vi "Steuerprogramm09-15.vi"() -> ()   [LabVIEW 2010]
uses:
  <vilib>/rvi/interface/nirviReadWriteControl/nirviReadWriteControl.xnode
  <vilib>/rvi/errors/niLvFpgaWhatHappensToTopLevelVI.ctl
  <vilib>/rvi/interface/common/niFpgaNodeNameForErrorReporting.ctl
  <vilib>/rvi/errors/niLvFpgaAdjustHostInterfaceError.vi
  gvbooleschRT.vi
  <vilib>/functionblocks/FB Core/FB Core.xnode
  <vilib>/functionblocks/Counter/Elapsed Timer/Elapsed Timer.vi
  <vilib>/functionblocks/NI_FunctionBlock Libraries.lvlib
  <vilib>/rvi/interface/nirviCloseFPGA/nirviCloseFPGA.xnode
  <vilib>/addons/control/pid/NI_PID_pid.lvlib
  C:/Users/HAGAR-IV/Desktop/Zeugs/Johnny/pertrasgc fpga/FPGA-Programm-10-14.vi
  C:/Users/HAGAR-IV/Desktop/Zeugs/markus/version feb 2012/FPGA Bitfiles/pertrasgcfpga2_FPGATarget_FPGA-Programm-10_16368CB6.lvbitx
  GVMWHorst.vi
  GVMethodenwechsel.vi
  GVHorstSP.vi
  GVZwangs.vi
  GVHK1Hz.vi
  GVHeizenLH.vi
  GVAIs.vi
  <vilib>/addons/control/pid/pid.llb/PID (DBL Array).vi
  GVTrapsMachs.vi
  GVaktuelleTDMS.vi
  GVECDs.vi
  GVZeitenZyklen.vi
  GVProbenvol.vi
  GVVentilposition.vi
  NiFpgaLv.dll
  <vilib>/Utility/error.llb/Error Cluster From Error Code.vi
  <vilib>/Instr/_visa.llb/VISA Configure Serial Port (Instr).vi
  <vilib>/rvi/interface/nirviMethod/nirviMethod.xnode
  GVChroms.vi
  <vilib>/FPGAPlugInAG/cRIO-9114/niLvFpga_Close_cRIO-9114.vi
panel:
  in  "An/Aus":bool
  in  "dargestellte Größe 3":i32(ring)=1 items=["U_WiderstandTrap1 [V]", "TemperaturTrap1 [°C]", "U_WiderstandTrap2 [V]", "TemperaturTrap2 [°C]", "TemperaturMach1 [°C]", "TemperaturMach2 [°C]", "PrC0", "PrC2C", "Regler18", "Regler17", "Regler19", "Regler16", "Regler15", "Regler14", "MFC2A", "MFC2B", "MFC2C", "PrC2A", "MFC2D", "MFC2E", "PrC2B"]
  in  "TafelWischen!":bool
  out "schnelleAnzeige":cluster{dbl[], dbl[]}(graph)
  in  "senden":bool
  in  "Schreibpuffer":string
  out "vomLicor":string
  in  "Licor":bool
  in  "SerielleKomm.":bool=TRUE
  in  "ECDSpeichern":bool=TRUE
  in  "HKSpeichern":bool
  in  "Methode speichern":bool
  in  "DetYMax":dbl=100.0
  in  "DetYMin":dbl
  in  "HK2YMax":dbl=100.0
  in  "HK2YMin":dbl
  in  "HK1YMax":dbl=100.0
  in  "HK1YMin":dbl
  out "ZyklusNummernGesamt":i32[](array[numeric])
  in  "Detektor":i32(ring) items=["ECD1", "ECD2"]
  out "Detektor":cluster{dbl[], dbl[]}[](graph)
  out "Zykluslängen [s]":dbl[](array[numeric])
  in  "veränderte Methode benutzen":bool
  in  "Methode verändern":bool
  in  "dargestellte Größe 2":i32(ring)=1 items=["T1-Trap1", "T1-Trap2", "T1-Stirling", "T1-PreCol1", "T1-PreCol2", "T1-MainCol1a", "T1-MainCol1b", "T1-MainCol2a", "T1-MainCol2b", "T1-Spare1", "T1-Spare2", "T1-Spare3", "T1-Spare4", "T1-Valve1B", "T1-Spare9", "T1-Valve1A", "T1-Spare10", "T1-TurboPump", "T1-StirlingPlatine", "T1-Spare5", "T1-Spare6", "T1-Spare7", "T1-Spare8", "F1-MFM1", "F1-MFM2", "P1-MethaneHP", "P1-MethaneLP", "P1-Vacuum", "TurboSpeed", "I1-MS-AC", "I1-Trap1", "I1-Trap2", "T2-ECD1a", "T2-ECD1b", "T2-ECD2a", "T2-ECD2b", "T2-Col1a", "T2-Col1b", "T2-Col2a", "T2-Col2b", "T2-Spare1", "T2-Spare2", "T2-Oven_a", "T2-Oven_b", "T2-Spare3", "T2-Spare4", "T2-Spare5", "F2-MFM0", "F2-MFM2A", "F2-MFM2B", "P2-N2O_HP", "P2-N2O_LP", "P2-CO2_HP", "P2-CO2_LP", "AI-Spare1", "AI-Spare2", "AI-Spare3", "AI-Spare4", "AI-Spare5", "AI-Spare6", "AI-Spare7", "AI-Spare8", "AI-Spare9", "AI-Spare10", "T0-DC/DC5", "I0-24V_M0", "I0-48V_M1", "I0-24V_M1", "I0-28V_M2", "T0-Drier", "T0-Spare2", "T0-Spare4", "T0-DC/DC7", "I0-20V_Laptop", "I0-28V_M1", "I0-24V_M2", "I0-12V_Licor", "T0-Spare1", "T0-Spare3", "T0-Spare5", "F0-MFM1", "TL-Licor_a", "P0-NitrogenHP", "P0-HeliumHP", "P0-Standard1HP", "P0-Standard2HP", "P0-Standard3HP", "AI-Spare11", "F0-MFM2", "TL-Licor_b", "P0-NitrogenLP", "P0-HeliumLP", "P0-Standard1LP", "P0-Standard2LP", "P0-Standard3LP", "AI-Spare12", "U_WiderstandTrap1 [V]", "TemperaturTrap1 [°C]", "U_WiderstandTrap2 [V]", "TemperaturTrap2 [°C]", "TemperaturMach1 [°C]", "TemperaturMach2 [°C]", "PrC0", "PrC2C", "Regler18", "Regler17", "Regler19", "Regler16", "Regler15", "Regler14", "MFC2A", "MFC2B", "MFC2C", "PrC2A", "MFC2D", "MFC2E", "PrC2B"]
  in  "Zeitachse2":i32(ring)=1 items=["Zykluszeit [s] Mod0", "Zykluszeit [s] Mod1", "Zykluszeit [s] Mod2A", "Zykluszeit [s] Mod2B"]
  out "Housekeeping2":cluster{dbl[], dbl[]}(graph)
  out "ZyklusNummern":i32[](array[numeric])
  in  "dargestellte Größe 1":i32(ring)=1 items=["T1-Trap1", "T1-Trap2", "T1-Stirling", "T1-PreCol1", "T1-PreCol2", "T1-MainCol1a", "T1-MainCol1b", "T1-MainCol2a", "T1-MainCol2b", "T1-Spare1", "T1-Spare2", "T1-Spare3", "T1-Spare4", "T1-Valve1B", "T1-Spare9", "T1-Valve1A", "T1-Spare10", "T1-TurboPump", "T1-StirlingPlatine", "T1-Spare5", "T1-Spare6", "T1-Spare7", "T1-Spare8", "F1-MFM1", "F1-MFM2", "P1-MethaneHP", "P1-MethaneLP", "P1-Vacuum", "TurboSpeed", "I1-MS-AC", "I1-Trap1", "I1-Trap2", "T2-ECD1a", "T2-ECD1b", "T2-ECD2a", "T2-ECD2b", "T2-Col1a", "T2-Col1b", "T2-Col2a", "T2-Col2b", "T2-Spare1", "T2-Spare2", "T2-Oven_a", "T2-Oven_b", "T2-Spare3", "T2-Spare4", "T2-Spare5", "F2-MFM0", "F2-MFM2A", "F2-MFM2B", "P2-N2O_HP", "P2-N2O_LP", "P2-CO2_HP", "P2-CO2_LP", "AI-Spare1", "AI-Spare2", "AI-Spare3", "AI-Spare4", "AI-Spare5", "AI-Spare6", "AI-Spare7", "AI-Spare8", "AI-Spare9", "AI-Spare10", "T0-DC/DC5", "I0-24V_M0", "I0-48V_M1", "I0-24V_M1", "I0-28V_M2", "T0-Drier", "T0-Spare2", "T0-Spare4", "T0-DC/DC7", "I0-20V_Laptop", "I0-28V_M1", "I0-24V_M2", "I0-12V_Licor", "T0-Spare1", "T0-Spare3", "T0-Spare5", "F0-MFM1", "TL-Licor_a", "P0-NitrogenHP", "P0-HeliumHP", "P0-Standard1HP", "P0-Standard2HP", "P0-Standard3HP", "AI-Spare11", "F0-MFM2", "TL-Licor_b", "P0-NitrogenLP", "P0-HeliumLP", "P0-Standard1LP", "P0-Standard2LP", "P0-Standard3LP", "AI-Spare12", "U_WiderstandTrap1 [V]", "TemperaturTrap1 [°C]", "U_WiderstandTrap2 [V]", "TemperaturTrap2 [°C]", "TemperaturMach1 [°C]", "TemperaturMach2 [°C]", "PrC0", "PrC2C", "Regler18", "Regler17", "Regler19", "Regler16", "Regler15", "Regler14", "MFC2A", "MFC2B", "MFC2C", "PrC2A", "MFC2D", "MFC2E", "PrC2B"]
  in  "Zeitachse1":i32(ring)=1 items=["Zykluszeit [s] Mod0", "Zykluszeit [s] Mod1", "Zykluszeit [s] Mod2A", "Zykluszeit [s] Mod2B"]
  out "Housekeeping1":cluster{dbl[], dbl[]}(graph)
  out "Big Ben, Methodenzeit, Zykluszeit0, Zykluszeit1, Zykluszeit2A, Zykluszeit2B":i32[](array[numeric])
  in  "global stop RT":bool
  in  "Methode":i32(ring) items=["Leer"]
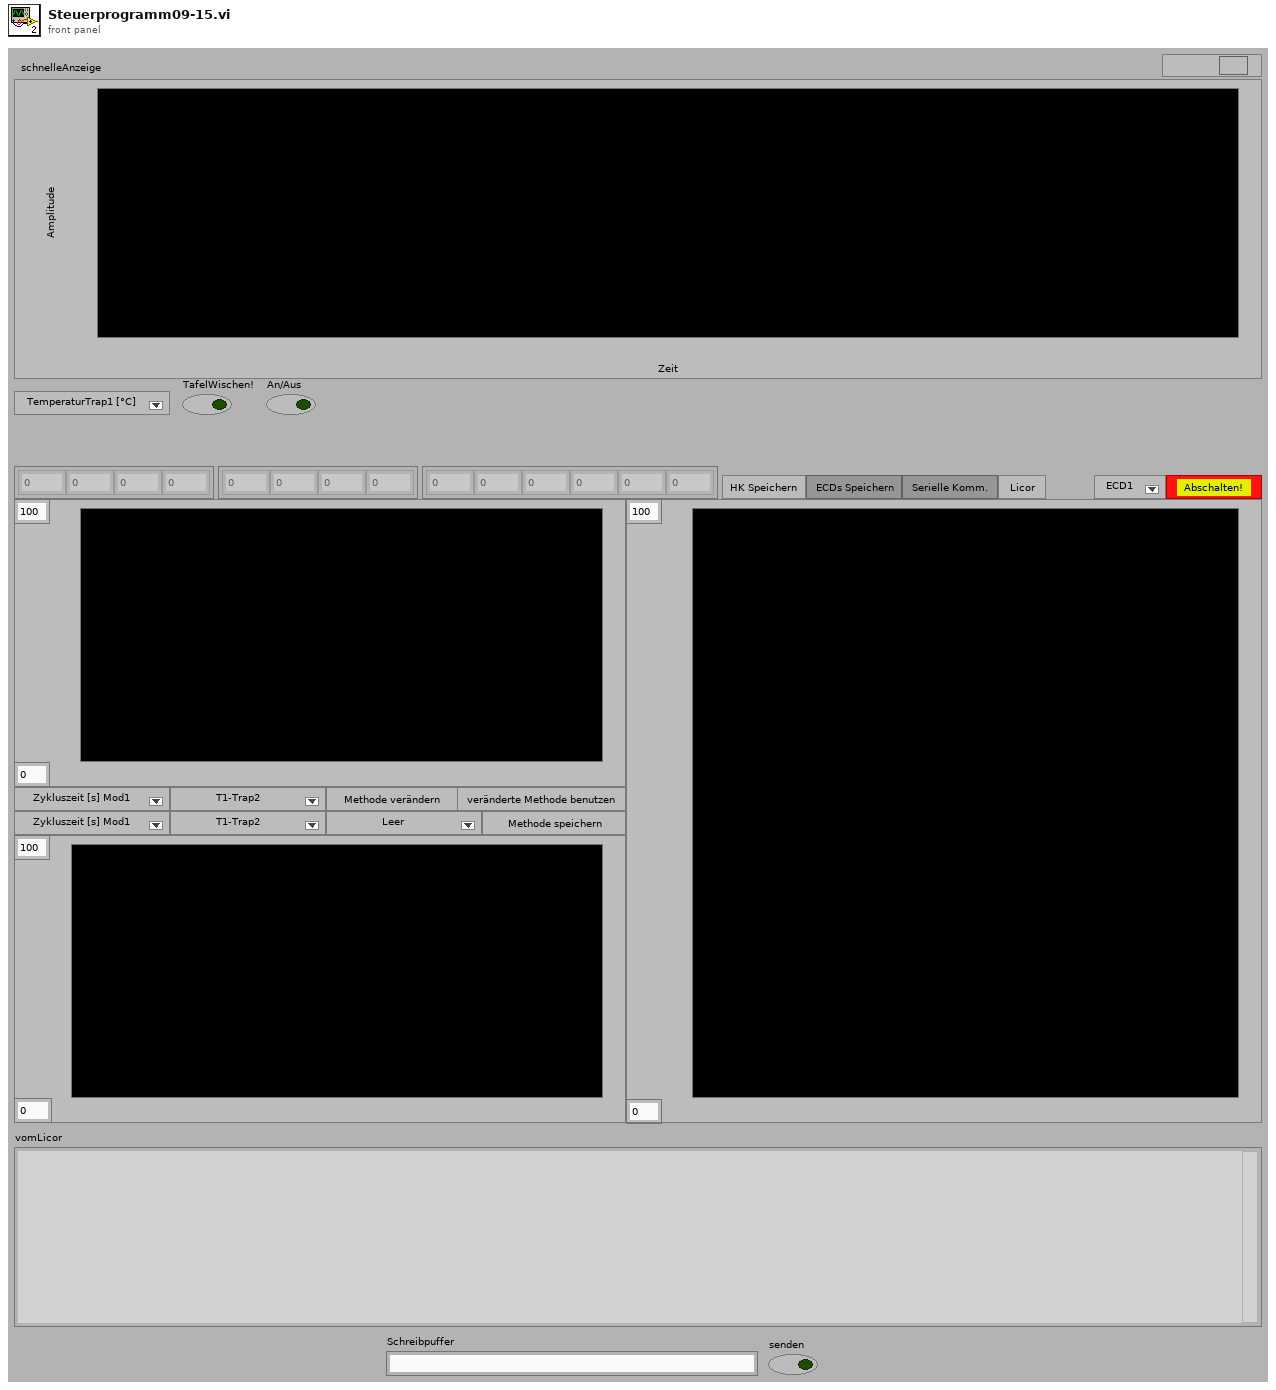
[diagram p1: front panel]
types:
  T1 = cluster{"Zykluslängen [s]":dbl[], "ZeitpktDIOsMod0":dbl[], "ZeitpktDIOsMod1":dbl[], "ZeitpktDIOsMod2A":dbl[], "ZeitpktDIOsMod2B":dbl[], "DIOsSPMod0":bool[][], "DIOsSPMod1":bool[][], "DIOsSPMod2A":bool[][], "DIOsSPMod2B":bool[][], "Mod0HorstZeitpkt":dbl[], "Mod1HorstZeitpkt":dbl[], "Mod2AHorstZeitpkt":dbl[], "Mod2BHorstZeitpkt":dbl[], "HorstSPMod0":dbl[][], "HorstSPMod1":dbl[][], "HorstSPMod2A":dbl[][], "HorstSPMod2B":dbl[][], "LangsameHeizungenSP":dbl[], "LHHeizen?":bool[], "ZPktFPGABoolesch":dbl[], "FPGABoolesch":bool[][], "ZeitpktFPGAPID":dbl[], "FPGAPID":cluster{"proportional gain (Kc)":fxp<+/-,16,8>, "integral gain (Kc*Ts/Ti)":fxp<+/-,16,8>, "derivative gain (Kc*Td/Ts)":fxp<+/-,16,8>}[][], "ZeitpktFPGAFixp":dbl[], "FPGAFixp":fxp<+/-,16,4>[][], "ZeitpktMach1":dbl[], "TempMach1":dbl[], "ZeitpktMach2":dbl[], "TempMach2":dbl[], "PIDs für \"träge\" Heizungen":cluster{"proportional gain (Kc)":dbl, "integral time (Ti, min)":dbl, "derivative time (Td, min)":dbl}[], "Zwangsbedingungen":dbl[][], "Dateien fürs MS schicken?":bool, "ZeitpunkteMPV":dbl[], "SPMPV":i32[], "ZeitpktMSa":dbl, "ZeitpktMSb":dbl, "Int.Start1":dbl, "Int.Stop1":dbl, "Int.Start2":dbl, "Int.Stop2":dbl, "Methodenname":string}[]
  T2 = cluster{"DIOsMod0Nr":i32[], "DIOsMod1Nr":i32[], "DIOsMod2ANr":i32[], "DIOsMod2BNr":i32[], "AIsLH":i32[], "Anzahl Horst/Modul":i32[], "Regler für den Probenfluß":i32, "StringSPvorgebenMod0":string[], "StringSPvorgebenMod1":string[], "StringSPvorgebenMod2A":string[], "StringSPvorgebenMod2B":string[], "StringMWAntwort0":string[], "StringMWAntwort1":string[], "StringMWAntwort2A":string[], "StringMWAntwort2B":string[], "UmrechnungHorst0":dbl[], "UmrechnungHorst1":dbl[], "UmrechnungHorst2A":dbl[], "UmrechnungHorst2B":dbl[], "StringMWabfragenMod0":string[], "StringMWabfragenMod1":string[], "StringMWabfragenMod2A":string[], "StringMWabfragenMod2B":string[], "Modul1/AI koeff":dbl[][], "Modul2/AI koeff":dbl[][], "Modul3/AI koeff":dbl[][], "Traps/MachsKoeff":dbl[][], "Modul1/AIsNamen":string[], "Modul2/AIsNamen":string[], "Modul3/AIsNamen":string[], "DIOsMod0Name":string[], "DIOsMod1Name":string[], "DIOsMod2AName":string[], "DIOsMod2BName":string[], "HorstMod0Name":string[], "HorstMod1Name":string[], "HorstMod2AName":string[], "HorstMod2BName":string[], "Startmethode":i32, "Dateiordner Housekeeping":path, "Dateiname Housekeeping":string, "DateiordnerECD1":path, "DateinameECD1":string, "DateiordnerECD2":path, "DateinameECD2":string, "NamenLangsameHeizungen":string[], "ModuleLH":i32[]}
  T3 = enum16{"open", "replace", "create", "open or create", "replace or create", "replace or create with confirmation"}
  T4 = cluster{"DIOsMod0Nr":i32[], "DIOsMod1Nr":i32[], "DIOsMod2ANr":i32[], "DIOsMod2BNr":i32[], "AIs für \"träge\" Heizungen":i32[], i32[], "AnschlüsseHorstMod0":enum8{"0", "1", "2", "3", "4", "5", "6", "7", "8"}[], "AnschlüsseHorstMod1":enum8{"0", "1", "2", "3", "4", "5", "6", "7", "8"}[], "AnschlüsseHorstMod2A":enum8{"0", "1", "2", "3", "4", "5", "6", "7", "8"}[], "AnschlüsseHorstMod2B":enum8{"0", "1", "2", "3", "4", "5", "6", "7", "8"}[], "StringSPvorgebenMod0":string[], "StringSPvorgebenMod1":string[], "StringSPvorgebenMod2A":string[], "StringSPvorgebenMod2B":string[], "StringMWAntwort0":string[], "StringMWAntwort1":string[], "StringMWAntwort2A":string[], "StringMWAntwort2B":string[], "UmrechnungHorst0":dbl[], "UmrechnungHorst1":dbl[], "UmrechnungHorst2A":dbl[], "UmrechnungHorst2B":dbl[], "StringMWabfragenMod0":string[], "StringMWabfragenMod1":string[], "StringMWabfragenMod2A":string[], "StringMWabfragenMod2B":string[], "Modul1/AI koeff":dbl[][], "Modul2/AI koeff":dbl[][], "Modul3/AI koeff":dbl[][], "Traps/MachKoeff":dbl[][], "AIsNamen":string[], "DIOsMod0Name":string[], "DIOsMod1Name":string[], "DIOsMod2AName":string[], "DIOsMod2BName":string[], "HorstMod0Name":string[], "HorstMod1Name":string[], "HorstMod2AName":string[], "HorstMod2BName":string[], "Startmethode":i32, "Dateiordner Housekeeping":path, "Dateiname Housekeeping":string, "DateiordnerECD1":path, "DateinameECD1":string, "DateiordnerECD2":path, "DateinameECD2":string}
  T5 = cluster{"Zykluslängen [s]":dbl[], "ZeitpktDIOsMod0":dbl[], "ZeitpktDIOsMod1":dbl[], "ZeitpktDIOsMod2A":dbl[], "ZeitpktDIOsMod2B":dbl[], "DIOsSPMod0":bool[][], "DIOsSPMod1":bool[][], "DIOsSPMod2A":bool[][], "DIOsSPMod2B":bool[][], "Mod0HorstZeitpkt":dbl[], "Mod1HorstZeitpkt":dbl[], "Mod2AHorstZeitpkt":dbl[], "Mod2BHorstZeitpkt":dbl[], "HorstSPMod0":dbl[][], "HorstSPMod1":dbl[][], "HorstSPMod2A":dbl[][], "HorstSPMod2B":dbl[][], "LangsameHeizungenSP":dbl[], "LHHeizen?":bool[], "ZPktFPGABoolesch":dbl[], "FPGABoolesch":bool[][], "ZeitpktFPGAPID":dbl[], "FPGAPID":cluster{"proportional gain (Kc)":fxp<+/-,16,8>, "integral gain (Kc*Ts/Ti)":fxp<+/-,16,8>, "derivative gain (Kc*Td/Ts)":fxp<+/-,16,8>}[][], "ZeitpktFPGAFixp":dbl[], "FPGAFixp":fxp<+/-,16,4>[][], "ZeitpktMach1":dbl[], "TempMach1":dbl[], "ZeitpktMach2":dbl[], "TempMach2":dbl[], "PIDs für \"träge\" Heizungen":cluster{"proportional gain (Kc)":dbl, "integral time (Ti, min)":dbl, "derivative time (Td, min)":dbl}[], "Zwangsbedingungen":dbl[][], "Text0 MS-Datei":string, "Info":string, "wie wird gespeichert?":u16, "Speicherlänge":string, "Dateien fürs MS schicken?":bool, "Pfad MS-Datei CRIO":path}[]
  T6 = cluster{"DIOsMod0Nr":i32[], "DIOsMod1Nr":i32[], "DIOsMod2ANr":i32[], "DIOsMod2BNr":i32[], "AIs für \"träge\" Heizungen":i32[], i32[], "AnschlüsseHorstMod0":enum8{"0", "1", "2", "3", "4", "5", "6", "7", "8"}[], "AnschlüsseHorstMod1":enum8{"0", "1", "2", "3", "4", "5", "6", "7", "8"}[], "AnschlüsseHorstMod2A":enum8{"0", "1", "2", "3", "4", "5", "6", "7", "8"}[], "AnschlüsseHorstMod2B":enum8{"0", "1", "2", "3", "4", "5", "6", "7", "8"}[], "StringSPvorgebenMod0":string[], "StringSPvorgebenMod1":string[], "StringSPvorgebenMod2A":string[], "StringSPvorgebenMod2B":string[], "StringMWAntwort0":string[], "StringMWAntwort1":string[], "StringMWAntwort2A":string[], "StringMWAntwort2B":string[], "UmrechnungHorst0":dbl[], "UmrechnungHorst1":dbl[], "UmrechnungHorst2A":dbl[], "UmrechnungHorst2B":dbl[], "StringMWabfragenMod0":string[], "StringMWabfragenMod1":string[], "StringMWabfragenMod2A":string[], "StringMWabfragenMod2B":string[], "Modul1/AI koeff":dbl[][], "Modul2/AI koeff":dbl[][], "Modul3/AI koeff":dbl[][], "Traps/MachKoeff":dbl[][], "AIsNamen":string[], "DIOsMod0Name":string[], "DIOsMod1Name":string[], "DIOsMod2AName":string[], "DIOsMod2BName":string[], "HorstMod0Name":string[], "HorstMod1Name":string[], "HorstMod2AName":string[], "HorstMod2BName":string[], "Startmethode":i32, "Dateiordner Housekeeping":path, "Dateiname Housekeeping":string}
  T7 = typedef "niFpgaNodeNameForErrorReporting.ctl" = enum16{"Open FPGA VI Reference", "Read/Write Control", "Invoke Method: Abort", "Invoke Method: Acknowledge IRQ", "Invoke Method: Download", "Invoke Method: FIFO.Configure", "Invoke Method: FIFO.Read", "Invoke Method: FIFO.Start", "Invoke Method: FIFO.Stop", "Invoke Method: FIFO.Write", "Invoke Method: Reset", "Invoke Method: Run", "Invoke Method: Wait on IRQ", "Close FPGA VI Reference"}
  T8 = typedef "niLvFpgaWhatHappensToTopLevelVI.ctl" = enum16{"top level VI scripted behind XNode", "top level VI inlined behind XNode"}
  T9 = cluster{"Zyklus1":i32, "Zeitachse1":i32, "dargestellte Größe 1":i32, "Zyklus2":i32, "Zeitachse2":i32, "dargestellte Größe 2":i32}
  T10 = cluster{"DIOsMod0Name":string[], "DIOsMod1Name":string[], "DIOsMod2AName":string[], "DIOsMod2BName":string[], "HorstMod0Name":string[], "HorstMod1Name":string[], "HorstMod2AName":string[], "HorstMod2BName":string[], "NamenLangsameHeizungen":string[]}
  T11 = cluster{"Dateiordner Housekeeping":path, "DateiordnerECD1":path, "DateiordnerECD2":path, "Dateiname Housekeeping":string, "DateinameECD1":string, "DateinameECD2":string, "tdms0":refnum<k34>, "tdms1":refnum<k34>, "tdms0":refnum<k34>, "tdms1":refnum<k34>, "tdms0":refnum<k34>, "tdms1":refnum<k34>}
  T12 = cluster{"Zykluslängen [s]":dbl[], "ZeitpktDIOsMod0":dbl[], "ZeitpktDIOsMod1":dbl[], "ZeitpktDIOsMod2A":dbl[], "ZeitpktDIOsMod2B":dbl[], "DIOsSPMod0":bool[][], "DIOsSPMod1":bool[][], "DIOsSPMod2A":bool[][], "DIOsSPMod2B":bool[][], "Mod0HorstZeitpkt":dbl[], "Mod1HorstZeitpkt":dbl[], "Mod2AHorstZeitpkt":dbl[], "Mod2BHorstZeitpkt":dbl[], "HorstSPMod0":dbl[][], "HorstSPMod1":dbl[][], "HorstSPMod2A":dbl[][], "HorstSPMod2B":dbl[][], "LangsameHeizungenSP":dbl[], "LHHeizen?":bool[], "ZPktFPGABoolesch":dbl[], "FPGABoolesch":bool[][], "ZeitpktFPGAPID":dbl[], "FPGAPID":cluster{"proportional gain (Kc)":fxp<+/-,16,8>, "integral gain (Kc*Ts/Ti)":fxp<+/-,16,8>, "derivative gain (Kc*Td/Ts)":fxp<+/-,16,8>}[][], "ZeitpktFPGAFixp":dbl[], "FPGAFixp":fxp<+/-,16,4>[][], "ZeitpktMach1":dbl[], "TempMach1":dbl[], "ZeitpktMach2":dbl[], "TempMach2":dbl[], "PIDs für \"träge\" Heizungen":cluster{"proportional gain (Kc)":dbl, "integral time (Ti, min)":dbl, "derivative time (Td, min)":dbl}[], "Zwangsbedingungen":dbl[][], "Dateien fürs MS schicken?":bool, "ZeitpunkteMPV":dbl[], "SPMPV":i32[], "ZeitpktMSa":dbl, "ZeitpktMSb":dbl, "Int.Start1":dbl, "Int.Stop1":dbl, "Int.Start2":dbl, "Int.Stop2":dbl, "Methodenname":string}
  T13 = cluster{"proportional gain (Kc)":fxp<+/-,16,8>, "integral gain (Kc*Ts/Ti)":fxp<+/-,16,8>, "derivative gain (Kc*Td/Ts)":fxp<+/-,16,8>}[][]
  T14 = cluster{"proportional gain (Kc)":dbl, "integral time (Ti, min)":dbl, "derivative time (Td, min)":dbl}[]
  T15 = cluster{"Heizen?LH[0]":bool, "Heizen?LH[1]":bool, "Heizen?LH[2]":bool, "Heizen?LH[3]":bool, "Heizen?LH[4]":bool, "Heizen?LH[5]":bool, "Heizen?LH[6]":bool, "Heizen?LH[7]":bool, "Heizen?LH[8]":bool, "Heizen?LH[9]":bool, "Heizen?LH[10]":bool, "Heizen?LH[11]":bool, "Heizen?LH[12]":bool, "Heizen?LH[13]":bool}
  T16 = cluster{"[0]":u32, "[1]":u32, "[2]":u32, "[3]":u32, "[4]":u32, "[5]":u32, "[6]":u32, "[7]":u32, "[8]":u32, "[9]":u32, "[10]":u32, "[11]":u32, "[12]":u32, "[13]":u32}
  T17 = cluster{cluster{"ZeitpktDIOsMod2B":dbl[]}[], cluster{"DIOsSPMod2B":bool[][]}[], cluster{"Mod2BHorstZeitpkt":dbl[]}[], cluster{"HorstSPMod2B":dbl[][]}[], "LHHeizen?":bool[], "ZPktFPGABoolesch":dbl[], "FPGABoolesch":bool[][], "ZeitpktFPGAPID":dbl[], "FPGAPID":cluster{"proportional gain (Kc)":fxp<+/-,16,8>, "integral gain (Kc*Ts/Ti)":fxp<+/-,16,8>, "derivative gain (Kc*Td/Ts)":fxp<+/-,16,8>}[][], "ZeitpktFPGAFixp":dbl[], "FPGAFixp":fxp<+/-,16,4>[][], "ZeitpktMach1":dbl[], "TempMach1":dbl[], "ZeitpktMach2":dbl[], "TempMach2":dbl[], "ZeitpunkteMPV":dbl[], "SPMPV":i32[]}
  T18 = cluster{"ZyklusNummern":i32[], "ZeilennummernDIOs":i32[], "ZwangsDIO?":cluster{bool[]}[], "ZeilennummernHorst":i32[], "ZwangsHorst?":cluster{bool[]}[], "ZeileFPGABoolesch":i32, "ZwangsFPGABoolesch?":bool[], "ZeileFPGAPID":i32, "ZeileFPGAFixp":i32, "ZeileMach1":i32, "ZeileMach2":i32, "ZeilennummerMPV":i32}
  T19 = cluster{"Zyklusnummern 0, 1, 2A, 2B":i32[], i32[], "ZwangsDIO?":cluster{bool[]}[], i32[], "ZwangsHorst?":cluster{bool[]}[], i32, "ZwangsFPGABoolesch?":bool[], i32, i32, i32, i32, "ZeilennummerMPV":i32}
  T20 = cluster{string[], string[], string[], dbl[], dbl[], dbl[]}
  T21 = cluster{"Befehle1":string[], "Befehle2":string[], "Befehle3":string[]}
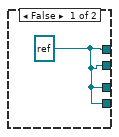
[diagram p2: hidden frame]
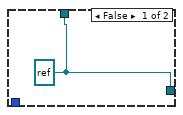
[diagram p3: hidden frame]
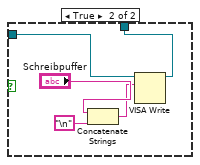
[diagram p6: hidden frame]
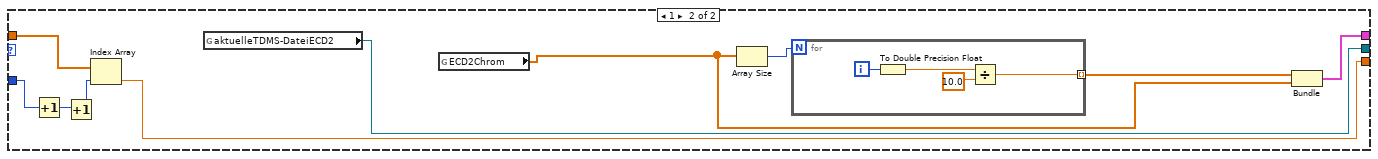
[diagram p14: hidden frame]
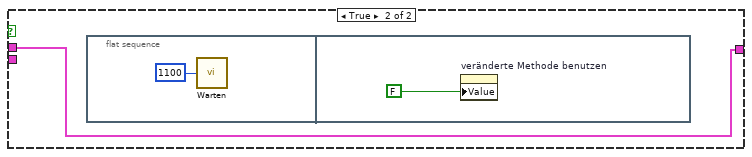
[diagram p15: hidden frame]
diagram:
  (unwired) T4 {"DIOsMod0Nr"=[], "DIOsMod1Nr"=[], "DIOsMod2ANr"=[], "DIOsMod2BNr"=[], "AIs für \"träge\" Heizungen"=[], [], "AnschlüsseHorstMod0"=[], "AnschlüsseHorstMod1"=[], "AnschlüsseHorstMod2A"=[], "AnschlüsseHorstMod2B"=[], "StringSPvorgebenMod0"=[], "StringSPvorgebenMod1"=[], "StringSPvorgebenMod2A"=[], "StringSPvorgebenMod2B"=[], "StringMWAntwort0"=[], "StringMWAntwort1"=[], "StringMWAntwort2A"=[], "StringMWAntwort2B"=[], "UmrechnungHorst0"=[], "UmrechnungHorst1"=[], "UmrechnungHorst2A"=[], "UmrechnungHorst2B"=[], "StringMWabfragenMod0"=[], "StringMWabfragenMod1"=[], "StringMWabfragenMod2A"=[], "StringMWabfragenMod2B"=[], "Modul1/AI koeff"=[], "Modul2/AI koeff"=[], "Modul3/AI koeff"=[], "Traps/MachKoeff"=[], "AIsNamen"=[], "DIOsMod0Name"=[], "DIOsMod1Name"=[], "DIOsMod2AName"=[], "DIOsMod2BName"=[], "HorstMod0Name"=[], "HorstMod1Name"=[], "HorstMod2AName"=[], "HorstMod2BName"=[], "Startmethode"=0, "Dateiordner Housekeeping"=path "", "Dateiname Housekeeping"="", "DateiordnerECD1"=path "", "DateinameECD1"="", "DateiordnerECD2"=path "", "DateinameECD2"=""} ("Einstellungen")
  (unwired) T5 [{"Zykluslängen [s]"=[180.0, 180.0, 180.0, 180.0], "ZeitpktDIOsMod0"=[0.0, 180.0], "ZeitpktDIOsMod1"=[0.0, 2.0, 15.0, 60.0, 61.0, 70.0, 80.0, 170.0, 180.0], "ZeitpktDIOsMod2A"=[0.0, 180.0], "ZeitpktDIOsMod2B"=[0.0, 60.0, 180.0], "DIOsSPMod0"=[[FALSE], [FALSE]], "DIOsSPMod1"=[[TRUE, TRUE, FALSE, TRUE, FALSE, TRUE, TRUE, TRUE, FALSE, FALSE, TRUE, FALSE, FALSE, FALSE, FALSE, FALSE, FALSE, TRUE], [TRUE, FALSE, FALSE, TRUE, FALSE, TRUE, TRUE, TRUE, FALSE, FALSE, TRUE, FALSE, FALSE, FALSE, FALSE, FALSE, FALSE, TRUE], [TRUE, FALSE, FALSE, FALSE, FALSE, TRUE, TRUE, FALSE, FALSE, FALSE, TRUE, FALSE, FALSE, FALSE, FALSE, FALSE, TRUE, TRUE], [TRUE, FALSE, FALSE, FALSE, FALSE, FALSE, TRUE, FALSE, FALSE, FALSE, TRUE, FALSE, FALSE, FALSE, FALSE, FALSE, TRUE, TRUE], [TRUE, FALSE, FALSE, FALSE, FALSE, FALSE, TRUE, FALSE, FALSE, FALSE, TRUE, FALSE, FALSE, FALSE, FALSE, FALSE, TRUE, TRUE], [TRUE, FALSE, FALSE, FALSE, FALSE, FALSE, TRUE, FALSE, FALSE, FALSE, TRUE, FALSE, FALSE, FALSE, FALSE, FALSE, TRUE, TRUE], [TRUE, FALSE, FALSE, FALSE, FALSE, FALSE, TRUE, FALSE, FALSE, FALSE, TRUE, FALSE, FALSE, FALSE, FALSE, FALSE, FALSE, TRUE], [TRUE, FALSE, FALSE, FALSE, FALSE, FALSE, TRUE, FALSE, FALSE, FALSE, TRUE, FALSE, FALSE, FALSE, FALSE, FALSE, FALSE, TRUE], [TRUE, FALSE, FALSE, FALSE, FALSE, FALSE, TRUE, FALSE, FALSE, FALSE, TRUE, FALSE, FALSE, FALSE, FALSE, FALSE, FALSE, TRUE]], "DIOsSPMod2A"=[[FALSE], [FALSE]], "DIOsSPMod2B"=[[FALSE], [FALSE]], "Mod0HorstZeitpkt"=[0.0, 180.0], "Mod1HorstZeitpkt"=[0.0, 55.0, 75.0, 180.0], "Mod2AHorstZeitpkt"=[0.0, 20.0, 180.0], "Mod2BHorstZeitpkt"=[0.0, 380.0], "HorstSPMod0"=[[2.66], [2.66]], "HorstSPMod1"=[[1.9, 0.0, 1.2], [0.0, 0.0, 1.2], [1.9, 0.0, 1.2], [1.9, 0.0, 1.2]], "HorstSPMod2A"=[[300.0], [300.0], [300.0]], "HorstSPMod2B"=[[0.0], [0.0]], "LangsameHeizungenSP"=[60.0, 220.0, 120.0, 60.0, 110.0, 0.0], "LHHeizen?"=[FALSE, TRUE, TRUE, FALSE, TRUE, FALSE], "ZPktFPGABoolesch"=[0.0, 60.0, 75.0, 180.0], "FPGABoolesch"=[[FALSE, FALSE, FALSE, FALSE, TRUE, FALSE], [FALSE, FALSE, TRUE, FALSE, TRUE, FALSE], [FALSE, FALSE, FALSE, FALSE, TRUE, FALSE], [FALSE, FALSE, FALSE, FALSE, TRUE, FALSE]], "ZeitpktFPGAPID"=[0.0, 60.0, 180.0], "FPGAPID"=[[{"proportional gain (Kc)"=5.0, "integral gain (Kc*Ts/Ti)"=0.0, "derivative gain (Kc*Td/Ts)"=0.0}, {"proportional gain (Kc)"=1.0, "integral gain (Kc*Ts/Ti)"=1.66796875, "derivative gain (Kc*Td/Ts)"=0.0}, {"proportional gain (Kc)"=5.0, "integral gain (Kc*Ts/Ti)"=0.03515625, "derivative gain (Kc*Td/Ts)"=0.0234375}, {"proportional gain (Kc)"=1.0, "integral gain (Kc*Ts/Ti)"=1.66796875, "derivative gain (Kc*Td/Ts)"=0.0}], [{"proportional gain (Kc)"=5.0, "integral gain (Kc*Ts/Ti)"=0.0, "derivative gain (Kc*Td/Ts)"=0.0}, {"proportional gain (Kc)"=1.0, "integral gain (Kc*Ts/Ti)"=1.66796875, "derivative gain (Kc*Td/Ts)"=0.0}, {"proportional gain (Kc)"=5.0, "integral gain (Kc*Ts/Ti)"=0.03515625, "derivative gain (Kc*Td/Ts)"=0.0234375}, {"proportional gain (Kc)"=1.0, "integral gain (Kc*Ts/Ti)"=1.66796875, "derivative gain (Kc*Td/Ts)"=0.0}], [{"proportional gain (Kc)"=0.0, "integral gain (Kc*Ts/Ti)"=0.0, "derivative gain (Kc*Td/Ts)"=0.0}, {"proportional gain (Kc)"=0.0, "integral gain (Kc*Ts/Ti)"=0.0, "derivative gain (Kc*Td/Ts)"=0.0}, {"proportional gain (Kc)"=2.0, "integral gain (Kc*Ts/Ti)"=0.03125, "derivative gain (Kc*Td/Ts)"=0.01953125}, {"proportional gain (Kc)"=0.0, "integral gain (Kc*Ts/Ti)"=0.0, "derivative gain (Kc*Td/Ts)"=0.0}], [{"proportional gain (Kc)"=0.0, "integral gain (Kc*Ts/Ti)"=0.0, "derivative gain (Kc*Td/Ts)"=0.0}, {"proportional gain (Kc)"=0.0, "integral gain (Kc*Ts/Ti)"=0.0, "derivative gain (Kc*Td/Ts)"=0.0}, {"proportional gain (Kc)"=2.0, "integral gain (Kc*Ts/Ti)"=0.03125, "derivative gain (Kc*Td/Ts)"=0.01953125}, {"proportional gain (Kc)"=0.0, "integral gain (Kc*Ts/Ti)"=0.0, "derivative gain (Kc*Td/Ts)"=0.0}], [{"proportional gain (Kc)"=0.0, "integral gain (Kc*Ts/Ti)"=0.0, "derivative gain (Kc*Td/Ts)"=0.0}, {"proportional gain (Kc)"=0.0, "integral gain (Kc*Ts/Ti)"=0.0, "derivative gain (Kc*Td/Ts)"=0.0}, {"proportional gain (Kc)"=2.0, "integral gain (Kc*Ts/Ti)"=0.03125, "derivative gain (Kc*Td/Ts)"=0.01953125}, {"proportional gain (Kc)"=0.0, "integral gain (Kc*Ts/Ti)"=0.0, "derivative gain (Kc*Td/Ts)"=0.0}]], "ZeitpktFPGAFixp"=[0.0, 60.0, 75.0, 180.0], "FPGAFixp"=[[0.0, 0.0, 0.0, 0.0, 0.0, 0.0, 2.85009765625, 0.0], [4.59423828125, 4.599365234375, 1.699951171875, 0.0, 0.0, 0.0, 2.85009765625, 0.0], [0.0, 0.0, 0.0, 0.0, 0.0, 0.0, 2.85009765625, 0.0], [0.0, 0.0, 0.0, 0.0, 0.0, 0.0, 2.85009765625, 0.0]], "ZeitpktMach1"=[0.0, 1.0, 100.0, 101.0, 177.0, 178.0, 180.0], "TempMach1"=[50.0, 50.0, 50.0, 250.0, 250.0, 50.0, 50.0], "ZeitpktMach2"=[0.0, 0.0, 120.0], "TempMach2"=[0.0, 0.0, 0.0], "PIDs für \"träge\" Heizungen"=[{"proportional gain (Kc)"=1.0, "integral time (Ti, min)"=0.01, "derivative time (Td, min)"=0.0}, {"proportional gain (Kc)"=2.0, "integral time (Ti, min)"=1.0, "derivative time (Td, min)"=0.0}, {"proportional gain (Kc)"=4.0, "integral time (Ti, min)"=1.0, "derivative time (Td, min)"=0.0}, {"proportional gain (Kc)"=1.0, "integral time (Ti, min)"=0.01, "derivative time (Td, min)"=0.0}, {"proportional gain (Kc)"=2.0, "integral time (Ti, min)"=0.0, "derivative time (Td, min)"=0.0}, {"proportional gain (Kc)"=1.0, "integral time (Ti, min)"=0.01, "derivative time (Td, min)"=0.0}], "Zwangsbedingungen"=[[3.0, 4.0, 100.0, 23.0, 4.0, 200.0, 0.0, 0.0]], "Text0 MS-Datei"="text0", "Info"="info", "wie wird gespeichert?"=0, "Speicherlänge"="100", "Dateien fürs MS schicken?"=FALSE, "Pfad MS-Datei CRIO"=path "c:/"}] ("Eingang 2")
  (unwired) T6 {"DIOsMod0Nr"=[32], "DIOsMod1Nr"=[5, 6, 7, 10, 11, 14, 15, 16, 17, 18, 20, 23, 25, 26, 27, 28, 29, 30], "DIOsMod2ANr"=[33], "DIOsMod2BNr"=[34], "AIs für \"träge\" Heizungen"=[17, 6, 0, 19, 21, 23], [1, 3, 1, 1], "AnschlüsseHorstMod0"=[enum."1"], "AnschlüsseHorstMod1"=[enum."1", enum."1", enum."1"], "AnschlüsseHorstMod2A"=[enum."1"], "AnschlüsseHorstMod2B"=[enum."1"], "StringSPvorgebenMod0"=[":060A020121"], "StringSPvorgebenMod1"=[":060B020121", ":0618020121", ":060D020121"], "StringSPvorgebenMod2A"=[":0519010104"], "StringSPvorgebenMod2B"=[":060C020121 "], "StringMWAntwort0"=[":060A020121"], "StringMWAntwort1"=[":060B020121", ":0618020121", ":060D020121"], "StringMWAntwort2A"=[":0619020121"], "StringMWAntwort2B"=[":060C020121"], "UmrechnungHorst0"=[0.0003125], "UmrechnungHorst1"=[9.375e-05, 9.375e-05, 9.375e-05], "UmrechnungHorst2A"=[1.0], "UmrechnungHorst2B"=[9.375e-05], "StringMWabfragenMod0"=[":060A0401210120"], "StringMWabfragenMod1"=[":060B0401210120", ":06180401210120", ":060D0401210120"], "StringMWabfragenMod2A"=[":06190401210120"], "StringMWabfragenMod2B"=[":060C0401210120"], "Modul1/AI koeff"=[[-249.333, 111.873, 2.1471], [-249.333, 111.873, 2.1471], [-249.333, 111.873, 2.1471], [-249.333, 111.873, 2.1471], [-237.2852, -153.162, 6.0782], [-237.2852, -153.162, 6.0782], [-249.333, 111.873, 2.1471], [-249.333, 111.873, 2.1471], [-249.333, 111.873, 2.1471], [-249.333, 111.873, 2.1471], [-249.333, 111.873, 2.1471], [-249.333, 111.873, 2.1471], [-249.333, 111.873, 2.1471], [-249.333, 111.873, 2.1471], [-249.333, 111.873, 2.1471], [0.0, 1.0, 0.0], [-249.333, 111.873, 2.1471], [-249.333, 111.873, 2.1471], [-249.333, 111.873, 2.1471], [-249.333, 111.873, 2.1471], [-249.333, 111.873, 2.1471], [-249.333, 111.873, 2.1471], [-249.333, 111.873, 2.1471], [-249.333, 111.873, 2.1471], [0.0, 1.0, 0.0], [0.0, 1.0, 0.0], [0.0, 1.0, 0.0], [0.0, 1.0, 0.0], [0.0, 1.0, 0.0], [0.0, 1.0, 0.0], [0.0, 1.0, 0.0], [0.0, 1.0, 0.0]], "Modul2/AI koeff"=[[0.0, 1.0, 0.0], [0.0, 1.0, 0.0], [0.0, 1.0, 0.0], [0.0, 1.0, 0.0], [0.0, 1.0, 0.0], [0.0, 1.0, 0.0], [0.0, 1.0, 0.0], [0.0, 1.0, 0.0], [0.0, 1.0, 0.0], [0.0, 1.0, 0.0], [0.0, 1.0, 0.0], [0.0, 1.0, 0.0], [0.0, 1.0, 0.0], [0.0, 1.0, 0.0], [0.0, 1.0, 0.0], [0.0, 1.0, 0.0], [0.0, 1.0, 0.0], [0.0, 1.0, 0.0], [0.0, 1.0, 0.0], [0.0, 1.0, 0.0], [0.0, 1.0, 0.0], [0.0, 1.0, 0.0], [0.0, 1.0, 0.0], [0.0, 1.0, 0.0], [0.0, 1.0, 0.0], [0.0, 1.0, 0.0], [0.0, 1.0, 0.0], [0.0, 1.0, 0.0], [0.0, 1.0, 0.0], [0.0, 1.0, 0.0], [0.0, 1.0, 0.0], [0.0, 1.0, 0.0]], "Modul3/AI koeff"=[[0.0, 1.0, 0.0], [0.0, 1.0, 0.0], [0.0, 1.0, 0.0], [0.0, 1.0, 0.0], [0.0, 1.0, 0.0], [0.0, 1.0, 0.0], [0.0, 1.0, 0.0], [0.0, 1.0, 0.0], [0.0, 1.0, 0.0], [0.0, 1.0, 0.0], [0.0, 1.0, 0.0], [0.0, 1.0, 0.0], [0.0, 1.0, 0.0], [0.0, 1.0, 0.0], [0.0, 1.0, 0.0], [0.0, 1.0, 0.0], [0.0, 1.0, 0.0], [0.0, 1.0, 0.0], [0.0, 1.0, 0.0], [0.0, 1.0, 0.0], [0.0, 1.0, 0.0], [0.0, 1.0, 0.0], [0.0, 1.0, 0.0], [0.0, 1.0, 0.0], [0.0, 1.0, 0.0], [0.0, 1.0, 0.0], [0.0, 1.0, 0.0], [0.0, 1.0, 0.0], [0.0, 1.0, 0.0], [0.0, 1.0, 0.0], [0.0, 1.0, 0.0], [0.0, 1.0, 0.0]], "Traps/MachKoeff"=[[0.0, 1.0, 0.0], [-249.333, 111.873, 2.1471], [0.0, 1.0, 0.0], [-249.333, 111.873, 2.1471], [-237.2852, 153.1621, 6.0782], [-237.2852, 153.1621, 6.0782]], "AIsNamen"=["T-MainCol3", "T-Trap1", "T-Trap2", "T-Stirling", "T-PreCol1", "T-PreCol2", "T-MainCol1", "T-MainCol2", "T-T-Line2", "T-MI1", "T-MI2", "T-MI3", "T-MI4", "T-MI5", "T-MI6", "F-MFM1", "T-MainCol4", "T-BHorst1", "T-BHorst2", "T-BHorst3", "T-BHorst4", "T-Oven1", "T-Oven2", "T-T-Line1", "F-MFM2", "P-Me-HP", "P-Me-LP", "P-Vac", "Ref-Turbo", "I-MS-AC", "I-Trap1", "I-Trap2", "Mod2/AI0", "Mod2/AI1", "Mod2/AI2", "Mod2/AI3", "Mod2/AI4", "Mod2/AI5", "Mod2/AI6", "Mod2/AI7", "Mod2/AI8", "Mod2/AI9", "Mod2/AI10", "Mod2/AI11", "Mod2/AI12", "Mod2/AI13", "Mod2/AI14", "Mod2/AI15", "Mod2/AI16", "Mod2/AI17", "Mod2/AI18", "Mod2/AI19", "Mod2/AI20", "Mod2/AI21", "Mod2/AI22", "Mod2/AI23", "Mod2/AI24", "Mod2/AI25", "Mod2/AI26", "Mod2/AI27", "Mod2/AI28", "Mod2/AI29", "Mod2/AI30", "Mod2/AI31", "Mod3/AI0", "Mod3/AI1", "Mod3/AI2", "Mod3/AI3", "Mod3/AI4", "Mod3/AI5", "Mod3/AI6", "Mod3/AI7", "Mod3/AI8", "Mod3/AI9", "Mod3/AI10", "Mod3/AI11", "Mod3/AI12", "Mod3/AI13", "Mod3/AI14", "Mod3/AI15", "Mod3/AI16", "Mod3/AI17", "Mod3/AI18", "Mod3/AI19", "Mod3/AI20", "Mod3/AI21", "Mod3/AI22", "Mod3/AI23", "Mod3/AI24", "Mod3/AI25", "Mod3/AI26", "Mod3/AI27", "Mod3/AI28", "Mod3/AI29", "Mod3/AI30", "Mod3/AI31"], "DIOsMod0Name"=["blindDIO0"], "DIOsMod1Name"=["on/off P-MS", "MS Start", "MS Stop", "FanMach1", "FanReserve", "Valve1A", "on/off PrePump", "Air-In", "on/off VacP2", "on/off VacP1", "S1D", "FanMach2", "S1C", "on/off Stirling", "S1B", "S1A", "Valve1B", "on/off Turbo"], "DIOsMod2AName"=["blindDIO2A"], "DIOsMod2BName"=["blindDIO2B"], "HorstMod0Name"=["MFC1B"], "HorstMod1Name"=["PressContr1A", "PressContr1B", "PressContr1C"], "HorstMod2AName"=["MFC1A"], "HorstMod2BName"=["PressContr1D"], "Startmethode"=0, "Dateiordner Housekeeping"=path "C:/data", "Dateiname Housekeeping"="test"} ("Einstellungen")
  (unwired) T6 {"DIOsMod0Nr"=[32], "DIOsMod1Nr"=[5, 6, 7, 10, 11, 14, 15, 16, 17, 18, 20, 23, 25, 26, 27, 28, 29, 30], "DIOsMod2ANr"=[33], "DIOsMod2BNr"=[34], "AIs für \"träge\" Heizungen"=[17, 6, 0, 19, 21, 23], [1, 3, 1, 1], "AnschlüsseHorstMod0"=[enum."1"], "AnschlüsseHorstMod1"=[enum."1", enum."1", enum."1"], "AnschlüsseHorstMod2A"=[enum."1"], "AnschlüsseHorstMod2B"=[enum."1"], "StringSPvorgebenMod0"=[":060A020121"], "StringSPvorgebenMod1"=[":060B020121", ":0618020121", ":060D020121"], "StringSPvorgebenMod2A"=[":0619020121"], "StringSPvorgebenMod2B"=[":060C020121"], "StringMWAntwort0"=[":060A020121"], "StringMWAntwort1"=[":060B020121", ":0618020121", ":060D020121"], "StringMWAntwort2A"=[":0619020121"], "StringMWAntwort2B"=[":060C020121"], "UmrechnungHorst0"=[0.0003125], "UmrechnungHorst1"=[9.375e-05, 9.375e-05, 9.375e-05], "UmrechnungHorst2A"=[0.046875], "UmrechnungHorst2B"=[9.375e-05], "StringMWabfragenMod0"=[":060A0401210120"], "StringMWabfragenMod1"=[":060B0401210120", ":06180401210120", ":060D0401210120"], "StringMWabfragenMod2A"=[":06190401210120"], "StringMWabfragenMod2B"=[":060C0401210120"], "Modul1/AI koeff"=[[-249.333, 111.873, 2.1471], [-249.333, 111.873, 2.1471], [-249.333, 111.873, 2.1471], [-249.333, 111.873, 2.1471], [-237.2852, -153.162, 6.0782], [-237.2852, -153.162, 6.0782], [-249.333, 111.873, 2.1471], [-249.333, 111.873, 2.1471], [-249.333, 111.873, 2.1471], [-249.333, 111.873, 2.1471], [-249.333, 111.873, 2.1471], [-249.333, 111.873, 2.1471], [-249.333, 111.873, 2.1471], [-249.333, 111.873, 2.1471], [-249.333, 111.873, 2.1471], [0.0, 1.0, 0.0], [-249.333, 111.873, 2.1471], [-249.333, 111.873, 2.1471], [-249.333, 111.873, 2.1471], [-249.333, 111.873, 2.1471], [-249.333, 111.873, 2.1471], [-249.333, 111.873, 2.1471], [-249.333, 111.873, 2.1471], [-249.333, 111.873, 2.1471], [0.0, 1.0, 0.0], [0.0, 1.0, 0.0], [0.0, 1.0, 0.0], [0.0, 1.0, 0.0], [0.0, 1.0, 0.0], [0.0, 1.0, 0.0], [0.0, 1.0, 0.0], [0.0, 1.0, 0.0]], "Modul2/AI koeff"=[[0.0, 1.0, 0.0], [0.0, 1.0, 0.0], [0.0, 1.0, 0.0], [0.0, 1.0, 0.0], [0.0, 1.0, 0.0], [0.0, 1.0, 0.0], [0.0, 1.0, 0.0], [0.0, 1.0, 0.0], [0.0, 1.0, 0.0], [0.0, 1.0, 0.0], [0.0, 1.0, 0.0], [0.0, 1.0, 0.0], [0.0, 1.0, 0.0], [0.0, 1.0, 0.0], [0.0, 1.0, 0.0], [0.0, 1.0, 0.0], [0.0, 1.0, 0.0], [0.0, 1.0, 0.0], [0.0, 1.0, 0.0], [0.0, 1.0, 0.0], [0.0, 1.0, 0.0], [0.0, 1.0, 0.0], [0.0, 1.0, 0.0], [0.0, 1.0, 0.0], [0.0, 1.0, 0.0], [0.0, 1.0, 0.0], [0.0, 1.0, 0.0], [0.0, 1.0, 0.0], [0.0, 1.0, 0.0], [0.0, 1.0, 0.0], [0.0, 1.0, 0.0], [0.0, 1.0, 0.0]], "Modul3/AI koeff"=[[0.0, 1.0, 0.0], [0.0, 1.0, 0.0], [0.0, 1.0, 0.0], [0.0, 1.0, 0.0], [0.0, 1.0, 0.0], [0.0, 1.0, 0.0], [0.0, 1.0, 0.0], [0.0, 1.0, 0.0], [0.0, 1.0, 0.0], [0.0, 1.0, 0.0], [0.0, 1.0, 0.0], [0.0, 1.0, 0.0], [0.0, 1.0, 0.0], [0.0, 1.0, 0.0], [0.0, 1.0, 0.0], [0.0, 1.0, 0.0], [0.0, 1.0, 0.0], [0.0, 1.0, 0.0], [0.0, 1.0, 0.0], [0.0, 1.0, 0.0], [0.0, 1.0, 0.0], [0.0, 1.0, 0.0], [0.0, 1.0, 0.0], [0.0, 1.0, 0.0], [0.0, 1.0, 0.0], [0.0, 1.0, 0.0], [0.0, 1.0, 0.0], [0.0, 1.0, 0.0], [0.0, 1.0, 0.0], [0.0, 1.0, 0.0], [0.0, 1.0, 0.0], [0.0, 1.0, 0.0]], "Traps/MachKoeff"=[[0.0, 1.0, 0.0], [-249.333, 111.873, 2.1471], [0.0, 1.0, 0.0], [-249.333, 111.873, 2.1471], [-237.2852, 153.1621, 6.0782], [-237.2852, 153.1621, 6.0782]], "AIsNamen"=["T-MainCol3", "T-Trap1", "T-Trap2", "T-Stirling", "T-PreCol1", "T-PreCol2", "T-MainCol1", "T-MainCol2", "T-T-Line2", "T-MI1", "T-MI2", "T-MI3", "T-MI4", "T-MI5", "T-MI6", "F-MFM1", "T-MainCol4", "T-BHorst1", "T-BHorst2", "T-BHorst3", "T-BHorst4", "T-Oven1", "T-Oven2", "T-T-Line1", "F-MFM2", "P-Me-HP", "P-Me-LP", "P-Vac", "Ref-Turbo", "I-MS-AC", "I-Trap1", "I-Trap2", "Mod2/AI0", "Mod2/AI1", "Mod2/AI2", "Mod2/AI3", "Mod2/AI4", "Mod2/AI5", "Mod2/AI6", "Mod2/AI7", "Mod2/AI8", "Mod2/AI9", "Mod2/AI10", "Mod2/AI11", "Mod2/AI12", "Mod2/AI13", "Mod2/AI14", "Mod2/AI15", "Mod2/AI16", "Mod2/AI17", "Mod2/AI18", "Mod2/AI19", "Mod2/AI20", "Mod2/AI21", "Mod2/AI22", "Mod2/AI23", "Mod2/AI24", "Mod2/AI25", "Mod2/AI26", "Mod2/AI27", "Mod2/AI28", "Mod2/AI29", "Mod2/AI30", "Mod2/AI31", "Mod3/AI0", "Mod3/AI1", "Mod3/AI2", "Mod3/AI3", "Mod3/AI4", "Mod3/AI5", "Mod3/AI6", "Mod3/AI7", "Mod3/AI8", "Mod3/AI9", "Mod3/AI10", "Mod3/AI11", "Mod3/AI12", "Mod3/AI13", "Mod3/AI14", "Mod3/AI15", "Mod3/AI16", "Mod3/AI17", "Mod3/AI18", "Mod3/AI19", "Mod3/AI20", "Mod3/AI21", "Mod3/AI22", "Mod3/AI23", "Mod3/AI24", "Mod3/AI25", "Mod3/AI26", "Mod3/AI27", "Mod3/AI28", "Mod3/AI29", "Mod3/AI30", "Mod3/AI31"], "DIOsMod0Name"=["blindDIO0"], "DIOsMod1Name"=["on/off P-MS", "MS Start", "MS Stop", "FanMach1", "FanReserve", "Valve1A", "on/off PrePump", "S1Reserve", "on/off VacP2", "on/off VacP1", "S1D", "FanMach2", "S1C", "on/off Stirling", "S1B", "S1A", "Valve1B", "on/off Turbo"], "DIOsMod2AName"=["blindDIO2A"], "DIOsMod2BName"=["blindDIO2B"], "HorstMod0Name"=["MFC1B"], "HorstMod1Name"=["PressContr1A", "PressContr1B", "PressContr1C"], "HorstMod2AName"=["MFC1A"], "HorstMod2BName"=["PressContr1D"], "Startmethode"=0, "Dateiordner Housekeeping"=path "C:/", "Dateiname Housekeeping"="test"} ("Einstellungen")
  n1 = Open/Create/Replace File(file path (use dialog)=path "c:/einstellungen.per" ("Datei (Dialog verwenden)"), operation (0:open)=T3."open" ("Operation (0:Öffnen)")) -> (refnum out=w11:refnum<file>)  [unwired: 4 in, 2 out]
  n2 = Read from Binary File(5:T2 {"DIOsMod0Nr"=[], "DIOsMod1Nr"=[], "DIOsMod2ANr"=[], "DIOsMod2BNr"=[], "AIsLH"=[], "Anzahl Horst/Modul"=[], "Regler für den Probenfluß"=0, "StringSPvorgebenMod0"=[], "StringSPvorgebenMod1"=[], "StringSPvorgebenMod2A"=[], "StringSPvorgebenMod2B"=[], "StringMWAntwort0"=[], "StringMWAntwort1"=[], "StringMWAntwort2A"=[], "StringMWAntwort2B"=[], "UmrechnungHorst0"=[], "UmrechnungHorst1"=[], "UmrechnungHorst2A"=[], "UmrechnungHorst2B"=[], "StringMWabfragenMod0"=[], "StringMWabfragenMod1"=[], "StringMWabfragenMod2A"=[], "StringMWabfragenMod2B"=[], "Modul1/AI koeff"=[], "Modul2/AI koeff"=[], "Modul3/AI koeff"=[], "Traps/MachsKoeff"=[], "Modul1/AIsNamen"=[], "Modul2/AIsNamen"=[], "Modul3/AIsNamen"=[], "DIOsMod0Name"=[], "DIOsMod1Name"=[], "DIOsMod2AName"=[], "DIOsMod2BName"=[], "HorstMod0Name"=[], "HorstMod1Name"=[], "HorstMod2AName"=[], "HorstMod2BName"=[], "Startmethode"=0, "Dateiordner Housekeeping"=path "", "Dateiname Housekeeping"="", "DateiordnerECD1"=path "", "DateinameECD1"="", "DateiordnerECD2"=path "", "DateinameECD2"="", "NamenLangsameHeizungen"=[], "ModuleLH"=[]} ("Einstellungen"), 11:w11) -> (2:w9:T2, 3:w10:refnum<file>)  [unwired: 4 in, 2 out]
  n3 = Close File(refnum=w10) -> ()  [unwired: 1 in, 2 out]
  n4 = flat-sequence {
    tunnel: [w158] -> w39
    tunnel: [w85] -> w38
    tunnel: [w183] -> w36
    tunnel: [w180] -> w35
    tunnel: [w182] -> w34
    tunnel: [w174] -> w33
    tunnel: [w181] -> w32
    tunnel: [w89] -> w31
    tunnel: [w173] -> w30
    tunnel: [w172] -> w29
    tunnel: [w165] -> w28
    tunnel: [w92] -> w27
    tunnel: [w62] -> w26
    tunnel: [w179] -> w25
    tunnel: [w171] -> w24
    tunnel: [w170] -> w23
    tunnel: [w161] -> w22
    tunnel: [w160] -> w21
    tunnel: [w159] -> w20
    tunnel: [w157] -> w19
    tunnel: [w156] -> w18
    tunnel: [w155] -> w17
    tunnel: [w152] -> w16
    tunnel: [w134] -> w15
    tunnel: w9 -> [w88]
    tunnel: [w132] -> w14
    tunnel: w3 -> [w133]
    tunnel: [w85] -> w1
    tunnel: w39 -> [w244]
    tunnel: w38 -> [w320]
    tunnel: [w244] -> w37
    tunnel: w36 -> [_]
    tunnel: w35 -> [w275]
    tunnel: w34 -> [w274]
    tunnel: w33 -> [w276]
    tunnel: w32 -> [w273]
    tunnel: w31 -> [w248]
    tunnel: w30 -> [w243]
    tunnel: w29 -> [w238]
    tunnel: w28 -> [w235]
    tunnel: w27 -> [w236]
    tunnel: w26 -> [w239]
    tunnel: w25 -> [w318]
    tunnel: w24 -> [w246]
    tunnel: w23 -> [w319]
    tunnel: w22 -> [w316]
    tunnel: w21 -> [w315]
    tunnel: w20 -> [w314]
    tunnel: w19 -> [w313]
    tunnel: w18 -> [w312]
    tunnel: w17 -> [w311]
    tunnel: w16 -> [w265]
    tunnel: w15 -> [w247]
    tunnel: w14 -> [w234]
    tunnel: w3 -> [w233]
    tunnel: w1 -> [w231]
    tunnel: w37 -> [w1174]
    frame #0 {
      w44 = 0.0 ("Probenvol.1")
      w51 = dbl[] [-1.0] ("ECD1MW")
      w52 = FALSE ("ECD1Empfangen?")
      w42 = string[] ["U_WiderstandTrap1 [V]", "TemperaturTrap1 [°C]", "U_WiderstandTrap2 [V]", "TemperaturTrap2 [°C]", "TemperaturMach1 [°C]", "TemperaturMach2 [°C]"]
      w177 = string[] ["Big Ben [s]", "Methodenzeit [s]", "Zykluszeit [s] Mod0", "Zykluszeit [s] Mod1", "Zykluszeit [s] Mod2A", "Zykluszeit [s] Mod2B"]
      w166 = FALSE ("Undefinierte Werte möglich")
      w168 = FALSE ("global stop RT")
      n5 = Unbundle(w88) -> ("DIOsMod0Nr"=w72:i32[], "DIOsMod1Nr"=w71:i32[], "DIOsMod2ANr"=w70:i32[], "DIOsMod2BNr"=w69:i32[], "AIsLH"=w59:i32[], "Anzahl Horst/Modul"=w62:i32[], "Regler für den Probenfluß"=w132:i32, "StringSPvorgebenMod0"=w131:string[], "StringSPvorgebenMod1"=w130:string[], "StringSPvorgebenMod2A"=w129:string[], "StringSPvorgebenMod2B"=w128:string[], "StringMWAntwort0"=w127:string[], "StringMWAntwort1"=w126:string[], "StringMWAntwort2A"=w125:string[], "StringMWAntwort2B"=w124:string[], "UmrechnungHorst0"=w123:dbl[], "UmrechnungHorst1"=w122:dbl[], "UmrechnungHorst2A"=w121:dbl[], "UmrechnungHorst2B"=w120:dbl[], "StringMWabfragenMod0"=w119:string[], "StringMWabfragenMod1"=w118:string[], "StringMWabfragenMod2A"=w117:string[], "StringMWabfragenMod2B"=w116:string[], "Modul1/AI koeff"=w115:dbl[][], "Modul2/AI koeff"=w114:dbl[][], "Modul3/AI koeff"=w113:dbl[][], "Traps/MachsKoeff"=w112:dbl[][], "Modul1/AIsNamen"=w111:string[], "Modul2/AIsNamen"=w110:string[], "Modul3/AIsNamen"=w109:string[], "DIOsMod0Name"=w107:string[], "DIOsMod1Name"=w106:string[], "DIOsMod2AName"=w105:string[], "DIOsMod2BName"=w104:string[], "HorstMod0Name"=w103:string[], "HorstMod1Name"=w102:string[], "HorstMod2AName"=w101:string[], "HorstMod2BName"=w100:string[], "Startmethode"=w85:i32, "Dateiordner Housekeeping"=w99:path, "Dateiname Housekeeping"=w98:string, "DateiordnerECD1"=w97:path, "DateinameECD1"=w96:string, "DateiordnerECD2"=w95:path, "DateinameECD2"=w94:string, "NamenLangsameHeizungen"=w93:string[], "ModuleLH"=w87:i32[])
      n6 = global write "gvbooleschRT.vi" "global stop RT"(w168) -> ()
      n7 = Decrement(x=w87) -> (x-1=w86:i32[])
      n8 = Multiply(x=w86, y=32) -> (x*y=w90:i32[])
      n9 = property on="dargestellte Größe 2" class="Ring (strict)"("AllowUndefVals"=w166) -> ()  [unwired: 2 in, 2 out]
      n10 = property on="Zeitachse2" class="Ring (strict)"("AllowUndefVals"=w166) -> ()  [unwired: 2 in, 2 out]
      n11 = property on="Zeitachse1" class="Ring (strict)"("AllowUndefVals"=w166) -> ()  [unwired: 2 in, 2 out]
      n12 = property on="dargestellte Größe 1" class="Ring (strict)"("AllowUndefVals"=w166) -> ()  [unwired: 2 in, 2 out]
      n13 = property on="Methode" class="Ring (strict)"("AllowUndefVals"=w166) -> ()  [unwired: 2 in, 2 out]
      n14 = property on="Methode" class="Ring (strict)"("Value"=w85) -> ()  [unwired: 2 in, 2 out]
      n15 = Add(x=w90, y=w59) -> (x+y=w89:i32[])
      n16 = Add Array Elements(numeric array=w62) -> (sum=w74:i32)
      n17 = for {
        tunnel: [w211] -> w175 mode=indexing
        tunnel: w133 -> [w212] mode=indexing
        n18 = Unbundle(w212) -> ("Methodenname"=w211:string)  [unwired: 40 out]
      }
      n19 = global write "GVProbenvol.vi" "Probenvol.2"(w44) -> ()
      n20 = global write "GVProbenvol.vi" "Probenvol.1"(w44) -> ()
      n21 = local write "global stop RT"(w168) -> ()
      n22 = Initialize Array(0.0 ("Element"), w74) -> (w73:dbl[])
      n23 = Initialize Array(-1.0, w74) -> (w76:dbl[])
      n24 = Initialize Array(-1.0 ("Element"), 96 ("Dimension")) -> (w56:dbl[])
      n25 = Initialize Array(-1.0 ("Element"), 6 ("Dimension")) -> (w55:dbl[])
      n26 = call "FPGA-Start.vi"() -> ("error out"=w183:errorcluster, "FPGA VI Reference Out"=w158:refnum<k20>)  [unwired: 2 in]
      n27 = global write "GVMWHorst.vi" "MWHorst"(w76) -> ()
      n28 = global write "GVHorstSP.vi" "HorstSP"(w73) -> ()
      n29 = global write "GVMethodenwechsel.vi" "Methodenwechsel?"(FALSE ("Methodenwechsel?")) -> ()
      n30 = global write "GVTrapsMachs.vi" "Traps/Machs"(w55) -> ()
      n31 = Build Array (concatenate)(w56, w55) -> (w54:dbl[])
      n32 = Build Array(w72, w71, w70, w69) -> (w68:i32[][])
      n33 = Build Array (concatenate)(w111, w110, w109) -> (w108:string[])
      n34 = global write "GVAIs.vi" "AIs"(w56) -> ()
      n35 = Array Size(array=w68) -> (size(s)=w67:i32[])
      n36 = local read "ECDSpeichern"() -> (w83:bool)
      n37 = property on="Methode" class="Ring (strict)"("Strings []"=w175) -> ()  [unwired: 2 in, 2 out]
      n38 = for {
        tunnel: w67 -> [w194] mode=indexing
        tunnel: [w191] -> w66 mode=indexing
        n39 = Initialize Array(FALSE, w194) -> (w192:bool[])
        n40 = Bundle(w192) -> (w191:cluster{bool[]})  [unwired: 1 in]
      }
      n41 = local read "HKSpeichern"() -> (w84:bool)
      n42 = Open/Create/Replace File(file path (use dialog)=path "c:/fromcriocmd.txt" ("Pfad MS-Datei CRIO"), operation (0:open)=T3."replace or create" ("Operation (0:Öffnen)")) -> (refnum out=w143:refnum<file>, error out=w142:errorcluster)  [unwired: 4 in, 1 out]
      n43 = Open/Create/Replace File(file path (use dialog)=path "c:/fromcriordy.txt" ("Dateipfad (Dialog verwenden)"), operation (0:open)=T3."replace or create" ("Operation (0:Öffnen)")) -> (refnum out=w137:refnum<file>, error out=w138:errorcluster)  [unwired: 4 in, 1 out]
      n44 = Write to Text File(file (use dialog)=w143, text="time=              \ncycle=   \ninfo=                                                                                                                                                      \nlength=   \ncmd=" ("Text0 MS-Datei"), error in=w142) -> (refnum out=w140:refnum<file>, error out=w139:errorcluster)  [unwired: 1 in, 1 out]
      n45 = case shown="True" w83 {
        tunnel: [w195 w204] -> w149
        tunnel: [w195 w203] -> w148
        tunnel: [w195 w202] -> w147
        tunnel: [w195 w201] -> w146
        tunnel: w97 -> [_ w200]
        tunnel: w96 -> [_ w199]
        tunnel: w95 -> [_ w198]
        tunnel: w94 -> [_ w197]
        tunnel: w85 -> [_ w196]
        frame False {
          w195 = refnum<k34> refnum ("tdms0")
        }
        frame True {
          n46 = call "TDMS0.vi"("Startmethode"=w196, "Dateiname"=w197, "Dateiordner"=w198) -> ("tdms1"=w201:refnum<k34>, "tdms0"=w202:refnum<k34>)
          n47 = call "TDMS0.vi"("Startmethode"=w196, "Dateiname"=w199, "Dateiordner"=w200) -> ("tdms1"=w203:refnum<k34>, "tdms0"=w204:refnum<k34>)
          n48 = global write "GVaktuelleTDMS.vi" "aktuelleTDMS-DateiECD1"(w204) -> ()
          n49 = global write "GVaktuelleTDMS.vi" "aktuelleTDMS-DateiECD2"(w202) -> ()
        }
      }
      n50 = global write "GVZwangs.vi" "ZwangsDIO!"(w66) -> ()
      n51 = global write "GVZwangs.vi" "ZwangsDIO?"(w66) -> ()
      n52 = Close File(refnum=w137, error in=w138) -> (path=w171:path)  [unwired: 1 out]
      n53 = Array Size(array=w59) -> (size(s)=w58:i32)
      n54 = case shown="True" w84 {
        tunnel: [w205 w210] -> w151
        tunnel: [w205 w209] -> w150
        tunnel: w99 -> [_ w208]
        tunnel: w98 -> [_ w207]
        tunnel: w85 -> [_ w206]
        frame False {
          w205 = refnum<k34> refnum ("tdms1")
        }
        frame True {
          n55 = call "TDMS0.vi"("Startmethode"=w206, "Dateiname"=w207, "Dateiordner"=w208) -> ("tdms1"=w209:refnum<k34>, "tdms0"=w210:refnum<k34>)
          n56 = global write "GVaktuelleTDMS.vi" "aktuelleTDMS-DateiHK"(w210) -> ()
        }
      }
      n57 = for {
        tunnel: w62 -> [w189] mode=indexing
        tunnel: [w186] -> w61 mode=indexing
        tunnel: [w184] -> w60 mode=indexing
        n58 = Initialize Array(0.0 ("Element"), w189) -> (w187:dbl[])
        n59 = Initialize Array(FALSE, w189) -> (w185:bool[])
        n60 = Bundle(w187) -> (w186:cluster{dbl[]})  [unwired: 1 in]
        n61 = Bundle(w185) -> (w184:cluster{bool[]})  [unwired: 1 in]
      }
      n62 = Close File(refnum=w140, error in=w139) -> (path=w134:path)  [unwired: 1 out]
      n63 = Initialize Array(FALSE, 6 ("Dimension")) -> (w63:bool[])
      n64 = Initialize Array(FALSE, w58) -> (w53:bool[])
      n65 = global write "GVZwangs.vi" "ZwangsFPGABoolesch?"(w63) -> ()
      n66 = global write "GVZwangs.vi" "ZwangsFPGABoolesch!"(w63) -> ()
      n67 = global write "GVZwangs.vi" "ZwangsLangsameH?"(w53) -> ()
      n68 = global write "GVZwangs.vi" "ZwangsLangsameH!"(w53) -> ()
      n69 = global write "GVZwangs.vi" "ZwangsHorst!"(w61) -> ()
      n70 = global write "GVZwangs.vi" "ZwangsHorst?"(w60) -> ()
      n71 = global write "GVHK1Hz.vi" "Mod1Mod2Mod3/AITrapsMachs1Hz"(w54) -> ()
      n72 = global write "GVHeizenLH.vi" "Heizen?LH"(w53) -> ()
      n73 = global write "GVECDs.vi" "ECD1Empfangen?"(w52) -> ()
      n74 = global write "GVECDs.vi" "ECD2Empfangen?"(w52) -> ()
      n75 = global write "GVECDs.vi" "ECD2MW"(w51) -> ()
      n76 = global write "GVECDs.vi" "ECD1MW"(w51) -> ()
      n77 = Build Array (concatenate)(w103, w102, w101, w100) -> (w41:string[])
      n78 = Build Array (concatenate)(w131, w130, w129, w128) -> (w182:string[])
      n79 = Build Array (concatenate)(w119, w118, w117, w116) -> (w180:string[])
      n80 = Initialize Array(0.0 ("Element"), 6 ("Dimension")) -> (w48:dbl[])
      n81 = global write "GVZeitenZyklen.vi" "Big Ben, Methodenzeit, Zykluszeit0, Zykluszeit1, Zykluszeit2A, Zykluszeit2B"(w48) -> ()
      n82 = Build Array (concatenate)(w127, w126, w125, w124) -> (w181:string[])
      n83 = Add Array Elements(numeric array=w62) -> (sum=w165:i32)
      n84 = Build Array (concatenate)(w123, w122, w121, w120) -> (w174:dbl[])
      n85 = Build Array (concatenate)(w42, w41) -> (w40:string[])
      n86 = Initialize Array(0, 4 ("Dimension")) -> (w45:i32[])
      n87 = Split 1D Array(array=w177, index=2 ("Index")) -> (second subarray=w169:string[])  [unwired: 1 out]
      n88 = property on="Zeitachse1" class="Ring (strict)"("Strings []"=w169) -> ()  [unwired: 2 in, 2 out]
      n89 = property on="Zeitachse2" class="Ring (strict)"("Strings []"=w169) -> ()  [unwired: 2 in, 2 out]
      n90 = global write "GVZeitenZyklen.vi" "ZyklusNummernGesamt"(w45) -> ()
      n91 = global write "GVZeitenZyklen.vi" "ZyklusNummern"(w45) -> ()
      n92 = global write "GVVentilposition.vi" "Ventilposition"(1 ("Ventilposition")) -> ()
      n93 = Build Array (concatenate)(w108, w42, w41) -> (w167:string[])
      n94 = property on="dargestellte Größe 3" class="Ring (strict)"("Strings []"=w40) -> ()  [unwired: 2 in, 2 out]
      n95 = Index Array(array=w112, index (col)=2 ("Deaktivierter Index (Spalte)")) -> (element=w161:dbl[])  [unwired: 1 in]
      n96 = Index Array(array=w112, index (col)=1 ("Deaktivierter Index (Spalte)")) -> (element=w160:dbl[])  [unwired: 1 in]
      n97 = Index Array(array=w112, index (col)=0 ("Deaktivierter Index (Spalte)")) -> (element=w159:dbl[])  [unwired: 1 in]
      n98 = call "AIKoeffSortieren.vi"("Modul3/AI koeff"=w113, "Modul2/AI koeff"=w114, "Modul1/AI koeff"=w115) -> ("P0"=w155:dbl[], "P1"=w156:dbl[], "P2"=w157:dbl[])
      n99 = Build Cluster Array(w72, w71, w70, w69) -> (w173:cluster{"DIOsMod2BNr":i32[]}[])
      n100 = for {
        tunnel: w173 -> [w214] mode=indexing
        tunnel: [w215] -> w172 mode=indexing
        n101 = Unbundle(w214) -> ("DIOsMod2BNr"=w213:i32[])
        n102 = Array Size(array=w213) -> (size(s)=w215:i32)
      }
      n103 = property on="dargestellte Größe 1" class="Ring (strict)"("Strings []"=w167) -> ()  [unwired: 2 in, 2 out]
      n104 = property on="dargestellte Größe 2" class="Ring (strict)"("Strings []"=w167) -> ()  [unwired: 2 in, 2 out]
      n105 = Bundle("DIOsMod0Name"=w107, "DIOsMod1Name"=w106, "DIOsMod2AName"=w105, "DIOsMod2BName"=w104, "HorstMod0Name"=w103, "HorstMod1Name"=w102, "HorstMod2AName"=w101, "HorstMod2BName"=w100, "NamenLangsameHeizungen"=w93) -> (w170:T10)  [unwired: 1 in]
      n106 = Build Array (concatenate)(string[] ["Datei Nr.", "Zyklusnr. Mod0", "Zyklusnr. Mod1", "Zyklusnr. Mod2A", "Zyklusnr. Mod2B"], w177, w108, w42, w41, "Probenvolumen1", "Probenvolumen2") -> (w179:string[])
      n107 = Bundle("Dateiordner Housekeeping"=w99, "DateiordnerECD1"=w97, "DateiordnerECD2"=w95, "Dateiname Housekeeping"=w98, "DateinameECD1"=w96, "DateinameECD2"=w94, "tdms0"=w151, "tdms1"=w150, "tdms0"=w149, "tdms1"=w148, "tdms0"=w147, "tdms1"=w146) -> (w152:T11)  [unwired: 1 in]
      n108 = Array Size(array=w93) -> (size(s)=w92:i32)
    }
    frame #1 {
      w216 = dbl[] [-1.0]
      w291 = 0
      w266 = 0 ("Zyklusnummer1")
      n109 = while {
        shift-right: ["Methode"] -> _
        shift-left: w320 -> [w1169]
        stop <- w1171 stop-if-true
        n110 = call "Bis zum nächsten Vielfachen warten7"("Count(mSec)"=u32 1000) -> ()  [unwired: 1 out]
        n111 = Not Equal?(x=w1169, y="Methode") -> (x != y?=w1167:bool)
        n112 = global write "GVMethodenwechsel.vi" "Methodenwechsel?"(w1167) -> ()
        n113 = global read "gvbooleschRT.vi" "global stop RT"() -> (w1171:bool)
      }
      n114 = Add Array Elements(numeric array=w238) -> (sum=w237:i32)
      n115 = flat-sequence {
        frame #0 {
          n116 = call "Warten5"("Count(mSec)"=u32 1000) -> ()  [unwired: 1 out]
        }
        frame #1 {
          n117 = case shown="True" "Licor" {
            frame False {
            }
            frame True {
              w352 = i16 128 items=["Unknown"=-1, "RS485/Wire4"=0, "RS485/Wire2-EchoDTR"=1, "RS485/Wire2-CtrlDTR"=2, "RS485/Wire2-Auto"=3, "RS232/DTE"=128, "RS232/DCE"=129, "RS232/AUTO"=130] ("Serial Settings:Wire Mode")
              n118 = call-poly "VISA Configure Serial Port"("VISA resource name"=refnum<visa-resource-name> "ASRL1::INSTR") -> ("VISA resource name out"=w351:refnum<visa-resource-name>)  [unwired: 13 in, 1 out]
              n119 = property class="Instr"(reference=w351, "Wire Mode"=w352) -> (reference out=w350:refnum<visa-resource-name>)  [unwired: 1 in, 1 out]
              n120 = VISA Flush I/O Buffer(VISA resource name=w350) -> (VISA resource name out=w349:refnum<visa-resource-name>)  [unwired: 2 in, 1 out]
              n121 = while {
                tunnel: w349 -> [w361]
                shift-right: [w363] -> _
                shift-left: "xxx" -> [w365]
                tunnel: [w357] -> w354
                stop <- w366 stop-if-true
                n122 = property class="Instr"(reference=w361) -> (reference out=w360:refnum<visa-resource-name>, "Serial Settings:Number of Bytes at Serial Port"=w359:u32)  [unwired: 1 in, 1 out]
                n123 = call "Warten4"("Count(mSec)"=u32 500) -> ()  [unwired: 1 out]
                n124 = VISA Read(VISA resource name=w360, byte count=w359) -> (VISA resource name out=w358:refnum<visa-resource-name>, read buffer=w364:string)  [unwired: 1 in, 2 out]
                n125 = global read "gvbooleschRT.vi" "global stop RT"() -> (w366:bool)
                n126 = Concatenate Strings(w365, w364) -> (w363:string)
                "vomLicor" <- w363
                n127 = case shown="False" "senden" {
                  tunnel: w358 -> [w367 w369]
                  tunnel: [w367 w368] -> w357
                  frame False {
                  }
                  frame True {
                    n128 = Concatenate Strings("Schreibpuffer", "\n") -> (w370:string)
                    n129 = VISA Write(VISA resource name=w369, write buffer=w370) -> (VISA resource name out=w368:refnum<visa-resource-name>)  [unwired: 1 in, 2 out]
                  }
                }
              }
              n130 = VISA Close(VISA resource name=w354) -> ()  [unwired: 1 in, 1 out]
            }
          }
        }
      }
      n131 = Array Size(array=w248) -> (size(s)=w269:i32)
      n132 = Index Array(array=w233, index=w231) -> (element=w232:T12)
      n133 = while {
        stop <- w1155 stop-if-true
        w1149 = 10.0
        n134 = global read "GVTrapsMachs.vi" "Traps/Machs"() -> (w1145:dbl[])
        n135 = global read "GVAIs.vi" "AIs"() -> (w1146:dbl[])
        n136 = call "Warten2"("Count(mSec)"=u32 1000) -> ()  [unwired: 1 out]
        n137 = for {
          N: 9 -> [_]
          shift-right: [w1158] -> w1152
          shift-left: w1146 -> [w1159]
          shift-right: [w1156] -> w1150
          shift-left: w1145 -> [w1157]
          n138 = flat-sequence {
            tunnel: w1159 -> [w1166]
            tunnel: [w1165] -> w1158
            tunnel: w1157 -> [w1164]
            tunnel: [w1163] -> w1156
            frame #0 {
              n139 = call "Warten28"("Count(mSec)"=u32 100) -> ()  [unwired: 1 out]
            }
            frame #1 {
              n140 = global read "GVTrapsMachs.vi" "Traps/Machs"() -> (w1161:dbl[])
              n141 = global read "GVAIs.vi" "AIs"() -> (w1162:dbl[])
              n142 = Add(x=w1166, y=w1162) -> (x+y=w1165:dbl[])
              n143 = Add(x=w1161, y=w1164) -> (x+y=w1163:dbl[])
            }
          }
        }
        n144 = Divide(x=w1152, y=w1149) -> (x/y=w1151:dbl[])
        n145 = Divide(x=w1150, y=w1149) -> (x/y=w1148:dbl[])
        n146 = Build Array (concatenate)(w1151, w1148) -> (w1147:dbl[])
        n147 = global write "GVHK1Hz.vi" "Mod1Mod2Mod3/AITrapsMachs1Hz"(w1147) -> ()
        n148 = global read "gvbooleschRT.vi" "global stop RT"() -> (w1155:bool)
      }
      n149 = while {
        tunnel: w244 -> [w674]
        tunnel: w313 -> [w673]
        tunnel: w312 -> [w672]
        tunnel: w311 -> [w671]
        stop <- w675 stop-if-true
        n150 = call "AIsFIFORT.vi"("P0"=w671, "P1"=w672, "P2"=w673, "FPGA VI Reference In"=w674) -> ()  [unwired: 1 in]
        n151 = global read "gvbooleschRT.vi" "global stop RT"() -> (w675:bool)
      }
      n152 = Initialize Array(cluster{"output high":dbl, "output low":dbl} {"output high"=99999.0, "output low"=0.0} ("output range"), w269) -> (w249:cluster{"output high":dbl, "output low":dbl}[])
      n153 = while {
        tunnel: w244 -> [w676]
        tunnel: w316 -> [w680]
        tunnel: w315 -> [w678]
        tunnel: w314 -> [w677]
        stop <- w681 stop-if-true
        n154 = call "TrapsMachMitteln.vi"("Traps/MachKoeff0"=w677, "Traps/MachKoeff1"=w678, "Traps/MachKoeff2"=w680, "FPGA VI Reference In"=w676) -> ()  [unwired: 1 in]
        n155 = global read "gvbooleschRT.vi" "global stop RT"() -> (w681:bool)
        n156 = call "Bis zum nächsten Vielfachen warten16"("Count(mSec)"=u32 100) -> ()  [unwired: 1 out]
      }
      n157 = Initialize Array(-1 ("Element"), 4 ("Dimension")) -> (w240:i32[])
      n158 = while {
        tunnel: w319 -> [w787]
        shift-right: [w786] -> _
        shift-left: w233 -> [w764]
        tunnel: w249 -> [w785]
        tunnel: w248 -> [w784]
        tunnel: w244 -> [w783]
        tunnel: w247 -> [w782]
        tunnel: w246 -> [w781]
        shift-right: [w773] -> _
        shift-left: 0 -> [w780]
        tunnel: w244 -> [w779]
        tunnel: w243 -> [w778]
        shift-right: [w772] -> _
        shift-left: 0.0 -> [w777]
        shift-right: [w771] -> _
        shift-left: -1 -> [w776]
        shift-right: [w770] -> _
        shift-left: w240 -> [w775]
        tunnel: w239 -> [w765]
        tunnel: w238 -> [w766]
        tunnel: w237 -> [w767]
        tunnel: w236 -> [w768]
        tunnel: w235 -> [w769]
        tunnel: w234 -> [w774]
        shift-right: [w685] -> _
        shift-left: w232 -> [w684]
        i -> [w688]
        stop <- w788 stop-if-true
        w730 = FALSE
        w729 = 0.0
        w731 = 0  # ZeilennummerMPV
        w735 = cluster{dbl[], dbl[]} {[], []}
        w745 = dbl[] []
        w749 = 0  # ZeileMach2
        w750 = 0  # ZeileMach1
        w751 = 0  # ZeileFPGAFixp
        w752 = 0  # ZeileFPGAPID
        w753 = 0  # ZeileFPGABoolesch
        w754 = i32[] [0, 0, 0, 0]  # ZeilennummernHorst
        w755 = i32[] [0, 0, 0, 0]  # ZeilennummernDIOs
        n159 = local read "Methode"() -> (w687:i32)
        n160 = Index Array(array=w764, index=w687) -> (element=w686:T12)
        n161 = Unbundle(w684) -> ("Zykluslängen [s]"=w728:dbl[], "ZeitpktDIOsMod0"=w727:dbl[], "ZeitpktDIOsMod1"=w726:dbl[], "ZeitpktDIOsMod2A"=w725:dbl[], "ZeitpktDIOsMod2B"=w724:dbl[], "DIOsSPMod0"=w723:bool[][], "DIOsSPMod1"=w722:bool[][], "DIOsSPMod2A"=w721:bool[][], "DIOsSPMod2B"=w720:bool[][], "Mod0HorstZeitpkt"=w719:dbl[], "Mod1HorstZeitpkt"=w718:dbl[], "Mod2AHorstZeitpkt"=w717:dbl[], "Mod2BHorstZeitpkt"=w716:dbl[], "HorstSPMod0"=w715:dbl[][], "HorstSPMod1"=w714:dbl[][], "HorstSPMod2A"=w713:dbl[][], "HorstSPMod2B"=w712:dbl[][], "LangsameHeizungenSP"=w711:dbl[], "LHHeizen?"=w710:bool[], "ZPktFPGABoolesch"=w709:dbl[], "FPGABoolesch"=w708:bool[][], "ZeitpktFPGAPID"=w707:dbl[], "FPGAPID"=w706:T13, "ZeitpktFPGAFixp"=w705:dbl[], "FPGAFixp"=w704:fxp<+/-,16,4>[][], "ZeitpktMach1"=w703:dbl[], "TempMach1"=w702:dbl[], "ZeitpktMach2"=w701:dbl[], "TempMach2"=w700:dbl[], "PIDs für \"träge\" Heizungen"=w699:T14, "Zwangsbedingungen"=w698:dbl[][], "Dateien fürs MS schicken?"=w697:bool, "ZeitpunkteMPV"=w696:dbl[], "SPMPV"=w695:i32[], "ZeitpktMSa"=w694:dbl, "ZeitpktMSb"=w693:dbl, "Int.Start1"=w692:dbl, "Int.Stop1"=w691:dbl, "Int.Start2"=w690:dbl, "Int.Stop2"=w689:dbl)  [unwired: 1 out]
        "Zykluslängen [s]" <- w728
        n162 = Add(x=w775, y=1) -> (x+y=w739:i32[])
        n163 = Add(x=w776, y=1) -> (x+y=w761:i32)
        n164 = global read "GVaktuelleTDMS.vi" "aktuelleTDMS-DateiECD1"() -> (w737:refnum<k34>)
        n165 = global read "GVZwangs.vi" "ZwangsFPGABoolesch?"() -> (w742:bool[])
        n166 = global read "GVZeitenZyklen.vi" "ZyklusNummern"() -> (w738:i32[])
        n167 = global read "GVZwangs.vi" "ZwangsHorst?"() -> (w744:cluster{bool[]}[])
        n168 = global read "GVZwangs.vi" "ZwangsDIO?"() -> (w743:cluster{bool[]}[])
        n169 = while {
          tunnel: w766 -> [w940]
          tunnel: w769 -> [w938]
          tunnel: w768 -> [w937]
          tunnel: w765 -> [w939]
          tunnel: w767 -> [w936]
          tunnel: w698 -> [w928]
          stop <- w930 stop-if-true
          n170 = local read "Methode"() -> (w935:i32)
          n171 = global read "gvbooleschRT.vi" "global stop RT"() -> (w933:bool)
          n172 = case shown="True" "global stop RT" {
            frame False {
            }
            frame True {
              n173 = global write "gvbooleschRT.vi" "global stop RT"(TRUE ("global stop RT")) -> ()
            }
          }
          n174 = call "ZwangsbedingungenGV.vi"("AnzahlHorst"=w938, "AnzahlHorst/Modul"=w939, "AnzahlLH"=w937, "AnzahlDIOs/Modul"=w940, "AnzahlDIOs"=w936, "Zwangsbedingungen"=w928, "Methodennummer"=w935) -> ("Methodennummer"=w934:i32)  [unwired: 4 in]
          n175 = local read "veränderte Methode benutzen"() -> (w931:bool)
          n176 = global read "GVMethodenwechsel.vi" "Methodenwechsel?"() -> (w932:bool)
          n177 = local write "Methode"(w934) -> ()
          n178 = Compound Arithmetic op=OR(w933, w932, w931) -> (w930:bool)
          n179 = call "Bis zum nächsten Vielfachen warten10"("Count(mSec)"=u32 1000) -> ()  [unwired: 1 out]
        }
        n180 = while {
          tunnel: w784 -> [w851]
          tunnel: w785 -> [w852]
          tunnel: w783 -> [w848]
          tunnel: w711 -> [w842]
          tunnel: w699 -> [w841]
          stop <- w837 stop-if-true
          n181 = global read "GVAIs.vi" "AIs"() -> (w843:dbl[])
          n182 = call "Bis zum nächsten Vielfachen warten12"("Count(mSec)"=u32 100) -> ()  [unwired: 1 out]
          n183 = for {
            tunnel: w843 -> [w927]
            tunnel: w851 -> [w926] mode=indexing
            tunnel: [w925] -> w850 mode=indexing
            n184 = Index Array(array=w927, index=w926) -> (element=w925:dbl)
          }
          n185 = global read "gvbooleschRT.vi" "global stop RT"() -> (w840:bool)
          n186 = local read "veränderte Methode benutzen"() -> (w838:bool)
          n187 = global read "GVMethodenwechsel.vi" "Methodenwechsel?"() -> (w839:bool)
          n188 = call-poly <vilib>:"PID.vi"("output range"=w852, "PID gains"=w841, "process variable"=w850, "setpoint"=w842) -> ("output"=w849:dbl[])  [unwired: 6 in, 1 out]
          n189 = global read "GVHeizenLH.vi" "Heizen?LH"() -> (w844:bool[])
          n190 = Compound Arithmetic op=OR(w840, w839, w838) -> (w837:bool)
          n191 = To Unsigned Long Integer(number=w849) -> (unsigned 32bit integer=w846:u32[])
          n192 = Array To Cluster(array=w844) -> (cluster=w847:T15)
          n193 = Array To Cluster(array=w846) -> (cluster=w845:T16)
          n194 = xnode "Read/Write Control"("FPGA VI Reference In"=w848, "LHHeizen?"=w847, "LHPulse(us)"=w845) -> ()  [unwired: 1 in, 2 out]
        }
        n195 = while {
          tunnel: w787 -> [w1121]
          shift-right: [w1112] -> _
          shift-left: w686 -> [w1120]
          tunnel: w687 -> [w1118]
          shift-right: [w1110] -> w786
          shift-left: w764 -> [w1119]
          tunnel: [w1111] -> w685
          stop <- w1114 stop-if-true
          n196 = global read "GVMethodenwechsel.vi" "Methodenwechsel?"() -> (w1116:bool)
          n197 = global read "gvbooleschRT.vi" "global stop RT"() -> (w1115:bool)
          n198 = case shown="True" "Methode verändern" {
            tunnel: w1121 -> [_ w1143]
            tunnel: w1120 -> [w1140 w1142]
            tunnel: [w1140 w1141] -> w1112
            frame False {
            }
            frame True {
              n199 = call "methodeändern.vi"("Methode"=w1142, "Namen"=w1143) -> ("Methode"=w1141:T12)  [unwired: 1 in]
              n200 = property on="Methode verändern" class="Bool (strict)"("Value"=FALSE ("Methode verändern")) -> ()  [unwired: 2 in, 2 out]
            }
          }
          n201 = Compound Arithmetic op=OR(w1116, w1115, "veränderte Methode benutzen") -> (w1114:bool)
          n202 = case shown="True" "Methode speichern" {
            tunnel: w1112 -> [_ w1137]
            tunnel: w1119 -> [w1130 w1139]
            tunnel: w1118 -> [_ w1138]
            tunnel: [w1130 w1132] -> w1110
            frame False {
            }
            frame True {
              n203 = Replace Array Subset(array=w1139, new element=w1137, index=w1138) -> (w1132:T1)
              n204 = property on="Methode speichern" class="Bool (strict)"("Value"=FALSE ("Methode speichern")) -> ()  [unwired: 2 in, 2 out]
              n205 = Open/Create/Replace File(file path (use dialog)=path "c:/methoden.per" ("Dateipfad (Dialog verwenden)"), operation (0:open)=T3."replace" ("Operation (0:Öffnen)")) -> (refnum out=w1134:refnum<file>)  [unwired: 4 in, 2 out]
              n206 = Write to Binary File(file (use dialog)=w1134, data=w1132) -> (refnum out=w1131:refnum<file>)  [unwired: 4 in, 2 out]
              n207 = Close File(refnum=w1131) -> ()  [unwired: 1 in, 2 out]
            }
          }
          n208 = case shown="False" "veränderte Methode benutzen" {
            tunnel: w1112 -> [_ w1127]
            tunnel: [w1124 w1127] -> w1111
            tunnel: w1110 -> [w1126 _]
            frame False {
              n209 = local read "Methode"() -> (w1125:i32)
              n210 = Index Array(array=w1126, index=w1125) -> (element=w1124:T12)
            }
            frame True {
              n211 = flat-sequence {
                frame #0 {
                  n212 = call "Warten"("Count(mSec)"=u32 1100) -> ()  [unwired: 1 out]
                }
                frame #1 {
                  n213 = property on="veränderte Methode benutzen" class="Bool (strict)"("Value"=FALSE ("Methode verändern")) -> ()  [unwired: 2 in, 2 out]
                }
              }
            }
          }
          n214 = call "Bis zum nächsten Vielfachen warten8"("Count(mSec)"=u32 500) -> ()  [unwired: 1 out]
        }
        n215 = Build Cluster Array(w723, w722, w721, w720) -> (w759:cluster{"DIOsSPMod2B":bool[][]}[])
        n216 = Build Cluster Array(w715, w714, w713, w712) -> (w757:cluster{"HorstSPMod2B":dbl[][]}[])
        n217 = Bundle(w745, w745, w745, w745) -> (w746:cluster{dbl[], dbl[], dbl[], dbl[]})  [unwired: 1 in]
        n218 = Build Cluster Array(w727, w726, w725, w724) -> (w760:cluster{"ZeitpktDIOsMod2B":dbl[]}[])
        n219 = Build Cluster Array(w719, w718, w717, w716) -> (w758:cluster{"Mod2BHorstZeitpkt":dbl[]}[])
        n220 = Equal?(x=w688, y=0) -> (x = y?=w762:bool)
        n221 = while {
          shift-right: [w801] -> _
          shift-left: w730 -> [w805]
          shift-right: [w800] -> _
          shift-left: w729 -> [w804]
          shift-right: [w799] -> _
          shift-left: w730 -> [w803]
          shift-right: [w798] -> _
          shift-left: w729 -> [w802]
          tunnel: w774 -> [w797]
          tunnel: w692 -> [w792]
          tunnel: w691 -> [w791]
          tunnel: w690 -> [w790]
          tunnel: w689 -> [w789]
          stop <- w794 stop-if-true
          n222 = call "Integrieren.vi"("Integrieren1"=w805, "Integral1"=w804, "Integrieren2"=w803, "Integral2"=w802, "Int.Start1"=w792, "Int.Stop1"=w791, "Int.Start2"=w790, "HorstProbenflußNr."=w797, "Int.Stop2"=w789) -> ("Integrieren1"=w801:bool, "Integral1"=w800:dbl, "Integrieren2"=w799:bool, "Integral2"=w798:dbl)  [unwired: 7 in]
          n223 = global read "gvbooleschRT.vi" "global stop RT"() -> (w796:bool)
          n224 = local read "veränderte Methode benutzen"() -> (w793:bool)
          n225 = global read "GVMethodenwechsel.vi" "Methodenwechsel?"() -> (w795:bool)
          n226 = Compound Arithmetic op=OR(w796, w795, w793) -> (w794:bool)
          n227 = call "Bis zum nächsten Vielfachen warten9"("Count(mSec)"=u32 100) -> ()  [unwired: 1 out]
        }
        n228 = Bundle(w760, w759, w758, w757, "LHHeizen?"=w710, "ZPktFPGABoolesch"=w709, "FPGABoolesch"=w708, "ZeitpktFPGAPID"=w707, "FPGAPID"=w706, "ZeitpktFPGAFixp"=w705, "FPGAFixp"=w704, "ZeitpktMach1"=w703, "TempMach1"=w702, "ZeitpktMach2"=w701, "TempMach2"=w700, "ZeitpunkteMPV"=w696, "SPMPV"=w695) -> (w756:T17)  [unwired: 1 in]
        n229 = Bundle("ZyklusNummern"=w738, "ZeilennummernDIOs"=w755, "ZwangsDIO?"=w743, "ZeilennummernHorst"=w754, "ZwangsHorst?"=w744, "ZeileFPGABoolesch"=w753, "ZwangsFPGABoolesch?"=w742, "ZeileFPGAPID"=w752, "ZeileFPGAFixp"=w751, "ZeileMach1"=w750, "ZeileMach2"=w749, "ZeilennummerMPV"=w731) -> (w748:T18)  [unwired: 1 in]
        n230 = while "ZyklusSteuerung" {
          tunnel: w778 -> [w1038]
          tunnel: w779 -> [w1036]
          shift-right: [w1034] -> _
          shift-left: w748 -> [w1035]
          tunnel: w756 -> [w1037]
          stop <- w1030 stop-if-true
          n231 = call "ZyklussteuerungGV.vi"("Zeitpunkte/SPs"=w1037, "DIOsNummern"=w1038, "Schieberegister"=w1035, "FPGA VI Reference In"=w1036) -> ("Schieberegister"=w1034:T19)  [unwired: 2 in]
          n232 = global read "gvbooleschRT.vi" "global stop RT"() -> (w1032:bool)
          n233 = local read "veränderte Methode benutzen"() -> (w1031:bool)
          n234 = global read "GVMethodenwechsel.vi" "Methodenwechsel?"() -> (w1033:bool)
          n235 = Compound Arithmetic op=OR(w1033, w1032, w1031) -> (w1030:bool)
          n236 = call "Bis zum nächsten Vielfachen warten11"("Count(mSec)"=u32 100) -> ()  [unwired: 1 out]
        }
        n237 = while {
          shift-right: [w988] -> _
          shift-left: w746 -> [w995]
          shift-right: [w987] -> _
          shift-left: w746 -> [w994]
          shift-right: [w985] -> _
          shift-left: T9 {"Zyklus1"=0, "Zeitachse1"=0, "dargestellte Größe 1"=0, "Zyklus2"=0, "Zeitachse2"=0, "dargestellte Größe 2"=0} ("AnzeigeEinstellungen") -> [w993]
          tunnel: w728 -> [w963]
          shift-right: [w959] -> _
          shift-left: w737 -> [w958]
          shift-right: [w954] -> _
          shift-left: w735 -> [w956]
          shift-right: [w943] -> _
          shift-left: w735 -> [w955]
          shift-right: ["Detektor"] -> _
          shift-left: 0 ("Detektor") -> [w952]
          stop <- w999 stop-if-true
          w964 = 0.0 ("X-Achse.Bereich:Minimum")
          n238 = case shown="0, Default" "Detektor" {
            tunnel: [w1009 w1021] -> w954
            tunnel: w963 -> [w1008 w1023]
            tunnel: "Detektor" -> [w1003 w1017]
            tunnel: [w1007 w1022] -> w961
            tunnel: [w1006 w1020] -> w959
            frame 0, Default {
              n239 = Increment(x=w1003) -> (x+1=w1004:i32)
              n240 = Increment(x=w1004) -> (x+1=w1002:i32)
              n241 = Index Array(array=w1008, index=w1002) -> (element=w1007:dbl)
              n242 = global read "GVaktuelleTDMS.vi" "aktuelleTDMS-DateiECD1"() -> (w1006:refnum<k34>)
              n243 = global read "GVChroms.vi" "ECD1Chrom"() -> (w1005:dbl[])
              n244 = Array Size(array=w1005) -> (size(s)=w1011:i32)
              n245 = for {
                N: w1011 -> [_]
                tunnel: [w1012] -> w1010 mode=indexing
                i -> [w1015]
                n246 = To Double Precision Float(number=w1015) -> (double precision float=w1014:dbl)
                n247 = Divide(x=w1014, y=10.0) -> (x/y=w1012:dbl)
              }
              n248 = Bundle(w1010, "ECD1Chrom"=w1005) -> (w1009:cluster{dbl[], "ECD1Chrom":dbl[]})  [unwired: 1 in]
            }
            frame 1 {
              n249 = Increment(x=w1017) -> (x+1=w1018:i32)
              n250 = Increment(x=w1018) -> (x+1=w1016:i32)
              n251 = Index Array(array=w1023, index=w1016) -> (element=w1022:dbl)
              n252 = global read "GVaktuelleTDMS.vi" "aktuelleTDMS-DateiECD2"() -> (w1020:refnum<k34>)
              n253 = global read "GVChroms.vi" "ECD2Chrom"() -> (w1019:dbl[])
              n254 = Array Size(array=w1019) -> (size(s)=w1025:i32)
              n255 = for {
                N: w1025 -> [_]
                tunnel: [w1026] -> w1024 mode=indexing
                i -> [w1029]
                n256 = To Double Precision Float(number=w1029) -> (double precision float=w1028:dbl)
                n257 = Divide(x=w1028, y=10.0) -> (x/y=w1026:dbl)
              }
              n258 = Bundle(w1024, "ECD2Chrom"=w1019) -> (w1021:cluster{dbl[], "ECD2Chrom":dbl[]})  [unwired: 1 in]
            }
          }
          n259 = global read "GVZeitenZyklen.vi" "Big Ben, Methodenzeit, Zykluszeit0, Zykluszeit1, Zykluszeit2A, Zykluszeit2B"() -> (w946:dbl[])
          n260 = global read "GVMethodenwechsel.vi" "Methodenwechsel?"() -> (w997:bool)
          n261 = local read "veränderte Methode benutzen"() -> (w996:bool)
          n262 = global read "gvbooleschRT.vi" "global stop RT"() -> (w998:bool)
          n263 = global read "GVZeitenZyklen.vi" "ZyklusNummern"() -> (w966:i32[])
          "ZyklusNummern" <- w966
          n264 = Or(x=w997, y=w998) -> (x .or. y?=w1000:bool)
          n265 = To Long Integer(number=w946) -> (32bit integer=→"Big Ben, Methodenzeit, Zykluszeit0, Zykluszeit1, Zykluszeit2A, Zykluszeit2B":i32[])
          n266 = Or(x=w1000, y=w996) -> (x .or. y?=w999:bool)
          n267 = Subtract(x="HK1YMax", y="HK1YMin") -> (x-y=w979:dbl)
          n268 = Subtract(x="HK2YMax", y="HK2YMin") -> (x-y=w974:dbl)
          n269 = call "AnzeigeGV.vi"("veränderte Methode benutzen"=w996, "Zykluslängen [s]"=w963, "Cluster1"=w995, "Big Ben, Methodenzeit, Zykluszeit0, Zykluszeit1, Zykluszeit2A, Zykluszeit2B"=w946, "Zyklusnummern 0, 1, 2A, 2B"=w966, "Cluster2"=w994, "AnzeigeEinstellungen"=w993, "dargestellte Größe 1"="dargestellte Größe 1", "Zeitachse1"="Zeitachse1", "dargestellte Größe 2"="dargestellte Größe 2", "Zeitachse2"="Zeitachse2") -> ("Anzeige2"=→"Housekeeping2":cluster{dbl[], dbl[]}, "Cluster1"=w988:cluster{dbl[], dbl[], dbl[], dbl[]}, "x1Inkr"=w983:dbl, "Cluster2"=w987:cluster{dbl[], dbl[], dbl[], dbl[]}, "Anzeige1"=→"Housekeeping1":cluster{dbl[], dbl[]}, "AnzeigeEinstellungen"=w985:T9, "x2Max"=w947:dbl, "x2Inkr"=w982:dbl, "x1Max"=w948:dbl)  [unwired: 8 in]
          n270 = Divide(x=w979, y=10.0) -> (x/y=w977:dbl)
          n271 = Divide(x=w974, y=10.0) -> (x/y=w972:dbl)
          n272 = property on="Housekeeping1" class="XYGraph (strict)"("XScale.Minimum"=w964, "XScale.Maximum"=w948, "XScale.Increment"=w983, "YScale.Minimum"="HK1YMin", "YScale.Maximum"="HK1YMax", "YScale.Increment"=w977) -> ()  [unwired: 2 in, 2 out]
          n273 = property on="Housekeeping2" class="XYGraph (strict)"("XScale.Minimum"=w964, "XScale.Maximum"=w947, "XScale.Increment"=w982, "YScale.Minimum"="HK2YMin", "YScale.Maximum"="HK2YMax", "YScale.Increment"=w972) -> ()  [unwired: 2 in, 2 out]
          n274 = Subtract(x="DetYMax", y="DetYMin") -> (x-y=w969:dbl)
          n275 = global read "GVZeitenZyklen.vi" "ZyklusNummernGesamt"() -> (→"ZyklusNummernGesamt":i32[])
          n276 = Equal?(x=w959, y=w958) -> (x = y?=w957:bool)
          n277 = Divide(x=w961, y=20.0) -> (x/y=w962:dbl)
          n278 = Divide(x=w969, y=20.0) -> (x/y=w967:dbl)
          n279 = Equal?(x="Detektor", y=w952) -> (x = y?=w951:bool)
          n280 = Select(t=w955, s=w957, f=w956) -> (s? t:f=w950:cluster{dbl[], dbl[]})
          n281 = property on="Detektor" class="XYGraph (strict)"("XScale.Minimum"=w964, "XScale.Maximum"=w961, "XScale.Increment"=w962, "YScale.Minimum"="DetYMin", "YScale.Maximum"="DetYMax", "YScale.Increment"=w967) -> ()  [unwired: 2 in, 2 out]
          n282 = Select(t=w950, s=w951, f=cluster{dbl[], dbl[]} {[], []} ("s? t:f")) -> (s? t:f=w943:cluster{dbl[], dbl[]})
          n283 = Build Array(w954, w943) -> (→"Detektor":cluster{dbl[], "ECD2Chrom":dbl[]}[])
          n284 = call "Bis zum nächsten Vielfachen warten14"("Count(mSec)"=u32 1000) -> ()  [unwired: 1 out]
        }
        n285 = global read "GVZeitenZyklen.vi" "Big Ben, Methodenzeit, Zykluszeit0, Zykluszeit1, Zykluszeit2A, Zykluszeit2B"() -> (w734:dbl[])
        n286 = while "Zeit" {
          tunnel: w762 -> [w1059]
          tunnel: [w1054] -> w772
          tunnel: w777 -> [w1058]
          tunnel: [w1048] -> w771
          tunnel: w761 -> [w1049]
          tunnel: w728 -> [w1056]
          tunnel: w739 -> [w1043]
          tunnel: [w1040] -> w770
          i -> [w1062]
          stop <- w1045 stop-if-true
          n287 = Equal?(x=w1062, y=0) -> (x = y?=w1060:bool)
          n288 = And(x=w1059, y=w1060) -> (x .and. y?=w1064:bool)
          n289 = xnode "Elapsed Timer"("reset"=w1064) -> ("elapsed time (ms)"=w1067:i32)  [unwired: 2 in, 1 out]
          n290 = global read "gvbooleschRT.vi" "global stop RT"() -> (w1057:bool)
          n291 = global read "GVMethodenwechsel.vi" "Methodenwechsel?"() -> (w1044:bool)
          n292 = local read "veränderte Methode benutzen"() -> (w1047:bool)
          n293 = To Double Precision Float(number=w1067) -> (double precision float=w1066:dbl)
          n294 = Or(x=w1044, y=w1057) -> (x .or. y?=w1046:bool)
          n295 = Divide(x=w1066, y=1000.0) -> (x/y=w1054:dbl)
          n296 = Or(x=w1047, y=w1046) -> (x .or. y?=w1045:bool)
          n297 = Subtract(x=w1054, y=w1058) -> (x-y=w1053:dbl)
          n298 = for {
            tunnel: w1056 -> [w1070] mode=indexing
            tunnel: w1053 -> [w1071]
            tunnel: [w1069] -> w1055 mode=indexing
            tunnel: [w1068] -> w1052 mode=indexing
            n299 = Quotient & Remainder(x=w1071, y=w1070) -> (x-y*floor(x/y)=w1069:dbl, floor(x/y)=w1068:dbl)
          }
          n300 = Build Array (concatenate)(w1054, w1053, w1055) -> (w1042:dbl[])
          n301 = global write "GVZeitenZyklen.vi" "Big Ben, Methodenzeit, Zykluszeit0, Zykluszeit1, Zykluszeit2A, Zykluszeit2B"(w1042) -> ()
          n302 = To Long Integer(number=w1052) -> (32bit integer=w1041:i32[])
          n303 = global write "GVZeitenZyklen.vi" "ZyklusNummern"(w1041) -> ()
          n304 = Add(x=w1041, y=w1043) -> (x+y=w1040:i32[])
          n305 = Index Array(array=w1041, index=1 ("Index")) -> (element=w1050:i32)
          n306 = Add(x=w1050, y=w1049) -> (x+y=w1048:i32)
          n307 = global write "GVZeitenZyklen.vi" "ZyklusNummernGesamt"(w1040) -> ()
          n308 = call "Bis zum nächsten Vielfachen warten15"("Count(mSec)"=u32 50) -> ()  [unwired: 1 out]
        }
        n309 = Index Array(array=w734, index=3 ("Index")) -> (element=w732:dbl)
        n310 = while {
          tunnel: w782 -> [w809]
          tunnel: w781 -> [w808]
          tunnel: w697 -> [w823]
          shift-right: [w824] -> w773
          shift-left: w780 -> [w825]
          tunnel: w694 -> [w819]
          tunnel: w693 -> [w813]
          shift-right: [w810] -> _
          shift-left: w732 -> [w814]
          stop <- w826 stop-if-true
          n311 = global read "gvbooleschRT.vi" "global stop RT"() -> (w829:bool)
          n312 = local read "veränderte Methode benutzen"() -> (w827:bool)
          n313 = global read "GVMethodenwechsel.vi" "Methodenwechsel?"() -> (w828:bool)
          n314 = Compound Arithmetic op=OR(w829, w828, w827) -> (w826:bool)
          n315 = global read "GVZeitenZyklen.vi" "Big Ben, Methodenzeit, Zykluszeit0, Zykluszeit1, Zykluszeit2A, Zykluszeit2B"() -> (w821:dbl[])
          n316 = Index Array(array=w821, index=3 ("Index")) -> (element=w810:dbl)
          n317 = Greater Or Equal?(x=w810, y=w819) -> (x >= y?=w818:bool)
          n318 = Less?(x=w814, y=w819) -> (x < y?=w817:bool)
          n319 = Greater Or Equal?(x=w810, y=w813) -> (x >= y?=w816:bool)
          n320 = Less?(x=w814, y=w813) -> (x < y?=w815:bool)
          n321 = And(x=w816, y=w815) -> (x .and. y?=w812:bool)
          n322 = And(x=w818, y=w817) -> (x .and. y?=w807:bool)
          n323 = Or(x=w807, y=w812) -> (x .or. y?=w811:bool)
          n324 = And(x=w823, y=w811) -> (x .and. y?=w822:bool)
          n325 = case shown="True" w822 {
            tunnel: w825 -> [w831 w832]
            tunnel: [w831 w836] -> w824
            tunnel: w809 -> [_ w835]
            tunnel: w808 -> [_ w834]
            tunnel: w807 -> [_ w833]
            frame False {
            }
            frame True {
              n326 = call "MSDateienSchicken02-15.vi"("MSNummer"=w832, "MSa?"=w833, "Dateipfad:fromcriordy"=w834, "Dateipfad:fromcriocmd"=w835) -> ()  [unwired: 1 in]
              n327 = Increment(x=w832) -> (x+1=w836:i32)
            }
          }
          n328 = call "Bis zum nächsten Vielfachen warten13"("Count(mSec)"=u32 100 ("Zu wartende ms")) -> ()  [unwired: 1 out]
        }
        n329 = global read "gvbooleschRT.vi" "global stop RT"() -> (w788:bool)
      }
      n330 = case shown="True" "ECDSpeichern" {
        frame False {
        }
        frame True {
          w612 = dbl[] []
          n331 = global read "GVaktuelleTDMS.vi" "aktuelleTDMS-DateiECD1"() -> (w613:refnum<k34>)
          n332 = while {
            shift-right: [w621] -> _
            shift-left: w612 -> [w625]
            shift-right: [w614] -> _
            shift-left: w612 -> [w618]
            shift-right: [w620] -> _
            shift-left: w613 -> [w623]
            tunnel: w612 -> [w617]
            stop <- w630 stop-if-true
            n333 = call "Bis zum nächsten Vielfachen warten3"("Count(mSec)"=u32 500) -> ()  [unwired: 1 out]
            n334 = global read "GVaktuelleTDMS.vi" "aktuelleTDMS-DateiECD1"() -> (w620:refnum<k34>)
            n335 = global read "GVaktuelleTDMS.vi" "aktuelleTDMS-DateiECD2"() -> (w628:refnum<k34>)
            n336 = global read "GVECDs.vi" "ECD2MW"() -> (w615:dbl[])
            n337 = Build Array (concatenate)(w618, w615) -> (w619:dbl[])
            n338 = global read "GVECDs.vi" "ECD1MW"() -> (w624:dbl[])
            n339 = Build Array (concatenate)(w625, w624) -> (w622:dbl[])
            n340 = global read "gvbooleschRT.vi" "global stop RT"() -> (w630:bool)
            n341 = Equal?(x=w623, y=w620) -> (x = y?=w616:bool)
            n342 = TDMS Write(0:w620, 7:"ECD1", 9:w624) -> ()  [unwired: 3 in, 4 out]
            n343 = TDMS Write(0:w628, 7:"ECD2", 9:w615) -> ()  [unwired: 3 in, 4 out]
            n344 = Select(t=w622, s=w616, f=w617) -> (s? t:f=w621:dbl[])
            n345 = global write "GVChroms.vi" "ECD1Chrom"(w621) -> ()
            n346 = Select(t=w619, s=w616, f=w617) -> (s? t:f=w614:dbl[])
            n347 = global write "GVChroms.vi" "ECD2Chrom"(w614) -> ()
          }
        }
      }
      n348 = case shown="True" "HKSpeichern" {
        tunnel: w318 -> [_ w653]
        frame False {
        }
        frame True {
          n349 = while {
            tunnel: w653 -> [w667]
            stop <- w670 stop-if-true
            n350 = global read "GVZeitenZyklen.vi" "Big Ben, Methodenzeit, Zykluszeit0, Zykluszeit1, Zykluszeit2A, Zykluszeit2B"() -> (w658:dbl[])
            n351 = call "Bis zum nächsten Vielfachen warten2"("Count(mSec)"=u32 1000) -> ()  [unwired: 1 out]
            n352 = global read "GVZeitenZyklen.vi" "ZyklusNummernGesamt"() -> (w656:i32[])
            n353 = global read "GVHK1Hz.vi" "Mod1Mod2Mod3/AITrapsMachs1Hz"() -> (w662:dbl[])
            n354 = global read "GVZeitenZyklen.vi" "ZyklusNummern"() -> (w657:i32[])
            n355 = global read "GVProbenvol.vi" "Probenvol.1"() -> (w655:dbl)
            n356 = global read "GVProbenvol.vi" "Probenvol.2"() -> (w654:dbl)
            n357 = global read "GVaktuelleTDMS.vi" "aktuelleTDMS-DateiHK"() -> (w661:refnum<k34>)
            n358 = global read "GVMWHorst.vi" "MWHorst"() -> (w663:dbl[])
            n359 = Index Array(array=w656, index=1 ("Index")) -> (element=w659:i32)
            n360 = To Double Precision Float(number=w659) -> (double precision float=w665:dbl)
            n361 = To Double Precision Float(number=w657) -> (double precision float=w664:dbl[])
            n362 = global read "gvbooleschRT.vi" "global stop RT"() -> (w670:bool)
            n363 = Build Array (concatenate)(w665, w664, w658, w662, w663, w655, w654) -> (w666:dbl[])
            n364 = TDMS Write(0:w661, 1:enum16{"decimated", "interleaved"}."interleaved" ("Daten-Layout (0:dezimiert)"), 7:w667, 9:w666) -> ()  [unwired: 2 in, 4 out]
          }
        }
      }
      n365 = while {
        shift-right: [w323] -> _
        shift-left: w216 -> [w325]
        shift-right: [w322] -> _
        shift-left: w216 -> [w324]
        stop <- w327 stop-if-true
        n366 = call "Bis zum nächsten Vielfachen warten"("Count(mSec)"=u32 100) -> ()  [unwired: 1 out]
        n367 = global read "gvbooleschRT.vi" "global stop RT"() -> (w327:bool)
        n368 = case shown="True" "An/Aus" {
          tunnel: w325 -> [w329 w345]
          tunnel: w324 -> [w328 w344]
          tunnel: [w329 w338] -> w323
          tunnel: [w328 w337] -> w322
          frame False {
          }
          frame True {
            w341 = dbl[] [] ("t")
            n369 = global read "GVZeitenZyklen.vi" "Big Ben, Methodenzeit, Zykluszeit0, Zykluszeit1, Zykluszeit2A, Zykluszeit2B"() -> (w332:dbl[])
            n370 = global read "GVTrapsMachs.vi" "Traps/Machs"() -> (w335:dbl[])
            n371 = global read "GVMWHorst.vi" "MWHorst"() -> (w334:dbl[])
            n372 = Build Array (concatenate)(w335, w334) -> (w333:dbl[])
            n373 = Index Array(array=w333, index="dargestellte Größe 3") -> (element=w346:dbl)
            n374 = Build Array (concatenate)(w345, w346) -> (w339:dbl[])
            n375 = Index Array(array=w332, index=1 ("Index")) -> (element=w330:dbl)
            n376 = Build Array (concatenate)(w344, w330) -> (w340:dbl[])
            n377 = Bundle(w340, w339) -> (→"schnelleAnzeige":cluster{dbl[], dbl[]})  [unwired: 1 in]
            n378 = Select(t=w341, s="TafelWischen!", f=w339) -> (s? t:f=w338:dbl[])
            n379 = Select(t=w341, s="TafelWischen!", f=w340) -> (s? t:f=w337:dbl[])
          }
        }
      }
      n380 = Index Array(array=w239, index #1=0 ("Index"), index #2=1 ("Index"), index #3=2 ("Index"), index #4=3 ("Index")) -> (element #1=w280:i32, element #2=w279:i32, element #3=w282:i32, element #4=w281:i32)
      n381 = Add(x=w282, y=w281) -> (x+y=w278:i32)
      n382 = Build Array(w280, w279, w278) -> (w277:i32[])
      n383 = for {
        N: 1 -> [_]
        tunnel: w244 -> [w682]
        tunnel: [w682] -> w271
        n384 = call "Warten8"("Count(mSec)"=u32 100) -> ()  [unwired: 1 out]
      }
      n385 = Index Array(array=w277, index #1=0 ("Index"), index #2=1 ("Index")) -> (element #1=w298:i32, element #2=w296:i32)
      n386 = Split 1D Array(array=w274, index=w298) -> (first subarray=w305:string[], second subarray=w307:string[])
      n387 = Split 1D Array(array=w276, index=w298) -> (first subarray=w302:dbl[], second subarray=w306:dbl[])
      n388 = Split 1D Array(array=w275, index=w298) -> (first subarray=w295:string[], second subarray=w297:string[])
      n389 = call <vilib>:"Space Constant.vi"() -> ("String"=w222:string)
      n390 = Concatenate Strings("?SE0,GDATA" ("Schreibpuffer"), "\r") -> (w217:string)
      n391 = Add Array Elements(numeric array=w277) -> (sum=w287:i32)
      n392 = Split 1D Array(array=w306, index=w296) -> (first subarray=w301:dbl[], second subarray=w300:dbl[])
      n393 = Build Array(w222) -> (w221:string[])
      n394 = Split 1D Array(array=w307, index=w296) -> (first subarray=w304:string[], second subarray=w303:string[])
      n395 = Split 1D Array(array=w297, index=w296) -> (first subarray=w294:string[], second subarray=w293:string[])
      n396 = Initialize Array("x", 8 ("Dimension")) -> (w223:string[])
      n397 = global read "GVVentilposition.vi" "Ventilposition"() -> (w250:i32)
      n398 = Bundle(w305, w304, w303, w302, w301, w300) -> (w299:T20)  [unwired: 1 in]
      n399 = Initialize Array(0.0, 8 ("Dimension")) -> (w218:dbl[])
      n400 = Bundle(w295, w294, w293) -> (w292:cluster{string[], string[], string[]})  [unwired: 1 in]
      n401 = Bundle(w221, w221, w221) -> (w289:cluster{string[], string[], string[]})  [unwired: 1 in]
      n402 = Initialize Array(-1.0 ("Element"), w287) -> (w272:dbl[])
      n403 = Bundle(w291, w291, w291) -> (w290:cluster{i32, i32, i32})  [unwired: 1 in]
      n404 = case shown="True" "SerielleKomm." {
        tunnel: bool[] [TRUE, TRUE, TRUE, TRUE, TRUE, TRUE, TRUE, TRUE] -> [_ w387]
        tunnel: w223 -> [_ w386]
        tunnel: w299 -> [_ w385]
        tunnel: w298 -> [_ w384]
        tunnel: w296 -> [_ w383]
        tunnel: w292 -> [_ w382]
        tunnel: w290 -> [_ w381]
        tunnel: w289 -> [_ w380]
        tunnel: w276 -> [_ w379]
        tunnel: w273 -> [_ w378]
        tunnel: w272 -> [_ w377]
        tunnel: w271 -> [_ w374]
        tunnel: w250 -> [_ w376]
        tunnel: w218 -> [_ w375]
        tunnel: w217 -> [_ w373]
        frame False {
        }
        frame True {
          n405 = while {
            shift-right: [w557] -> _
            shift-left: w387 -> [w532]
            shift-right: [w540] -> _
            shift-left: w377 -> [w552]
            tunnel: w374 -> [w539]
            shift-right: [w530] -> _
            shift-left: w386 -> [w556]
            tunnel: w378 -> [w555]
            tunnel: w379 -> [w554]
            shift-right: [w542] -> _
            shift-left: w380 -> [w544]
            tunnel: w384 -> [w550]
            tunnel: w383 -> [w551]
            tunnel: w385 -> [w553]
            tunnel: w382 -> [w547]
            shift-right: [w546] -> _
            shift-left: w381 -> [w548]
            shift-right: [w536] -> _
            shift-left: w376 -> [w538]
            shift-right: [w533] -> _
            shift-left: w375 -> [w534]
            stop <- w541 stop-if-true
            n406 = for {
              tunnel: w532 -> [w561] mode=indexing
              tunnel: w534 -> [w558] mode=indexing
              tunnel: [w565] -> w533 mode=indexing
              tunnel: [w562] -> w531 mode=indexing
              n407 = global read "GVZeitenZyklen.vi" "Big Ben, Methodenzeit, Zykluszeit0, Zykluszeit1, Zykluszeit2A, Zykluszeit2B"() -> (w568:dbl[])
              n408 = Index Array(array=w568, index=0 ("Index")) -> (element=w566:dbl)
              n409 = Subtract(x=w566, y=w558) -> (x-y=w564:dbl)
              n410 = Greater?(x=w564, y=0.1) -> (0:w560:bool)
              n411 = Or(x=w561, y=w560) -> (x .or. y?=w559:bool)
              n412 = Select(t=w560, s=w560, f=w561) -> (s? t:f=w562:bool)
              n413 = Select(t=w566, s=w559, f=w558) -> (s? t:f=w565:dbl)
            }
            n414 = global read "GVHorstSP.vi" "HorstSP"() -> (w540:dbl[])
            n415 = call "Warten3"("Count(mSec)"=u32 10) -> ()  [unwired: 1 out]
            n416 = Not Equal?(x=w540, y=w552) -> (x != y?=w545:bool)
            n417 = call "NeueSP.vi"("Anzahl2"=w551, "Anzahl1"=w550, "AlteSP"=w552, 7:"NeueSP"=w540, "BefehleCluster"=w544, 10:"NeueSP"=w545, "ClusterFest"=w553) -> ("BefehleCluster"=w543:T21)  [unwired: 4 in]
            n418 = call "MPVSenden.vi"("Ventilposition"=w538, "FPGA VI Reference"=w539) -> ("Ventilposition"=w536:i32, "FPGA VI Reference"=w537:refnum<k20>)
            n419 = call "Senden.vi"("FPGA VI Reference In"=w537, "BefehlsCluster"=w543, "Senden?"=w531, "Abfragenr.Cluster"=w548, "AbfragenCluster"=w547) -> ("Senden?"=w549:bool[], "Abfragenr.Cluster"=w546:cluster{i32, i32, i32}, "BefehlsCluster"=w542:T21)  [unwired: 1 in]
            n420 = call "SeriellRead.vi"("SkalierungsfaktorHorst"=w554, "VorwortHorst"=w555, "Zwischenspeicher"=w556, "Senden?"=w549, "FPGA VI Reference In"=w537) -> ("Senden?"=w557:bool[], "Zwischenspeicher"=w530:string[])  [unwired: 5 in]
            n421 = global read "gvbooleschRT.vi" "global stop RT"() -> (w541:bool)
          }
          n422 = while {
            tunnel: w374 -> [w395]
            tunnel: w373 -> [w394]
            stop <- w397 stop-if-true
            n423 = String To Byte Array(string=w394) -> (unsigned byte array=w390:u8[])
            n424 = Join Numbers(hi=w390, lo=u8 5) -> ((hi.lo)=w392:u16[])
            n425 = call "Warten6"("Count(mSec)"=u32 500) -> ()  [unwired: 1 out]
            n426 = xnode "Invoke Method"("FPGA VI Reference In"=w395, "Data"=w392) -> ("FPGA VI Reference Out"=w391:refnum<k20>)  [unwired: 2 in, 2 out]
            n427 = Join Numbers(hi=w390, lo=u8 6) -> ((hi.lo)=w388:u16[])
            n428 = xnode "Invoke Method"("FPGA VI Reference In"=w391, "Data"=w388) -> ()  [unwired: 2 in, 3 out]
            n429 = global read "gvbooleschRT.vi" "global stop RT"() -> (w397:bool)
          }
        }
      }
      n430 = Unbundle(w265) -> ("Dateiordner Housekeeping"=w264:path, "DateiordnerECD1"=w262:path, "DateiordnerECD2"=w261:path, "Dateiname Housekeeping"=w263:string, "DateinameECD1"=w260:string, "DateinameECD2"=w259:string, "tdms0"=w258:refnum<k34>, "tdms1"=w257:refnum<k34>, "tdms0"=w256:refnum<k34>, "tdms1"=w255:refnum<k34>, "tdms0"=w254:refnum<k34>, "tdms1"=w253:refnum<k34>)
      n431 = local read "HKSpeichern"() -> (w229:bool)
      n432 = case shown="True" w229 {
        tunnel: w266 -> [_ w637]
        tunnel: w264 -> [_ w636]
        tunnel: w263 -> [_ w635]
        tunnel: w258 -> [_ w634]
        tunnel: w257 -> [_ w633]
        frame False {
        }
        frame True {
          n433 = while {
            shift-right: [w645] -> w632
            shift-left: w634 -> [w639]
            shift-right: [w649] -> w631
            shift-left: w633 -> [w641]
            shift-right: [w643] -> _
            shift-left: w637 -> [w650]
            tunnel: w635 -> [w646]
            tunnel: w636 -> [w647]
            stop <- w652 stop-if-true
            n434 = global read "GVZeitenZyklen.vi" "ZyklusNummernGesamt"() -> (w638:i32[])
            n435 = call "Bis zum nächsten Vielfachen warten5"("Count(mSec)"=u32 500) -> ()  [unwired: 1 out]
            n436 = Index Array(array=w638, index=1 ("Index")) -> (element=w643:i32)
            n437 = Greater?(x=w643, y=w650) -> (0:w642:bool)
            n438 = Select(t=w641, s=w642, f=w639) -> (s? t:f=w640:refnum<k34>)
            n439 = global write "GVaktuelleTDMS.vi" "aktuelleTDMS-DateiHK"(w640) -> ()
            n440 = local read "Methode"() -> (w648:i32)
            n441 = global read "gvbooleschRT.vi" "global stop RT"() -> (w652:bool)
            n442 = call "AktuelleTDMS.vi"("AktuelleTDMS"=w639, "Dateiordner"=w647, "NächsteTDMS"=w641, "NeuerZyklus?"=w642, "Methodennummer"=w648, "Zyklnumges"=w643, "Dateiname"=w646) -> ("AktuelleTDMS"=w645:refnum<k34>, "NächsteTDMS"=w649:refnum<k34>)  [unwired: 5 in, 2 out]
          }
          n443 = TDMS Close(11:w632) -> ()  [unwired: 1 in, 2 out]
          n444 = TDMS Close(11:w631) -> ()  [unwired: 1 in, 2 out]
        }
      }
      n445 = local read "ECDSpeichern"() -> (w227:bool)
      n446 = case shown="True" w227 {
        tunnel: w266 -> [_ w581]
        tunnel: w262 -> [_ w580]
        tunnel: w261 -> [_ w579]
        tunnel: w260 -> [_ w578]
        tunnel: w259 -> [_ w577]
        tunnel: w256 -> [_ w576]
        tunnel: w255 -> [_ w575]
        tunnel: w254 -> [_ w574]
        tunnel: w253 -> [_ w573]
        frame False {
        }
        frame True {
          n447 = while {
            shift-right: [w606] -> w572
            shift-left: w576 -> [w598]
            shift-right: [w607] -> w571
            shift-left: w575 -> [w600]
            shift-right: [w604] -> _
            shift-left: w581 -> [w608]
            tunnel: w580 -> [w603]
            tunnel: w578 -> [w602]
            stop <- w610 stop-if-true
            n448 = global read "GVZeitenZyklen.vi" "ZyklusNummernGesamt"() -> (w597:i32[])
            n449 = call "Bis zum nächsten Vielfachen warten4"("Count(mSec)"=u32 500) -> ()  [unwired: 1 out]
            n450 = Index Array(array=w597, index=2 ("Index")) -> (element=w604:i32)
            n451 = Greater?(x=w604, y=w608) -> (0:w601:bool)
            n452 = Select(t=w600, s=w601, f=w598) -> (s? t:f=w599:refnum<k34>)
            n453 = global write "GVaktuelleTDMS.vi" "aktuelleTDMS-DateiECD1"(w599) -> ()
            n454 = local read "Methode"() -> (w605:i32)
            n455 = global read "gvbooleschRT.vi" "global stop RT"() -> (w610:bool)
            n456 = call "AktuelleTDMS.vi"("AktuelleTDMS"=w598, "Dateiordner"=w603, "NächsteTDMS"=w600, "NeuerZyklus?"=w601, "Methodennummer"=w605, "Zyklnumges"=w604, "Dateiname"=w602) -> ("AktuelleTDMS"=w606:refnum<k34>, "NächsteTDMS"=w607:refnum<k34>)  [unwired: 5 in, 2 out]
          }
          n457 = while {
            shift-right: [w591] -> w570
            shift-left: w574 -> [w583]
            shift-right: [w592] -> w569
            shift-left: w573 -> [w585]
            shift-right: [w589] -> _
            shift-left: w581 -> [w593]
            tunnel: w579 -> [w588]
            tunnel: w577 -> [w587]
            stop <- w595 stop-if-true
            n458 = global read "GVZeitenZyklen.vi" "ZyklusNummernGesamt"() -> (w582:i32[])
            n459 = call "Bis zum nächsten Vielfachen warten6"("Count(mSec)"=u32 500) -> ()  [unwired: 1 out]
            n460 = Index Array(array=w582, index=3 ("Index")) -> (element=w589:i32)
            n461 = Greater?(x=w589, y=w593) -> (0:w586:bool)
            n462 = Select(t=w585, s=w586, f=w583) -> (s? t:f=w584:refnum<k34>)
            n463 = global write "GVaktuelleTDMS.vi" "aktuelleTDMS-DateiECD2"(w584) -> ()
            n464 = local read "Methode"() -> (w590:i32)
            n465 = global read "gvbooleschRT.vi" "global stop RT"() -> (w595:bool)
            n466 = call "AktuelleTDMS.vi"("AktuelleTDMS"=w583, "Dateiordner"=w588, "NächsteTDMS"=w585, "NeuerZyklus?"=w586, "Methodennummer"=w590, "Zyklnumges"=w589, "Dateiname"=w587) -> ("AktuelleTDMS"=w591:refnum<k34>, "NächsteTDMS"=w592:refnum<k34>)  [unwired: 5 in, 2 out]
          }
          n467 = TDMS Close(11:w571) -> ()  [unwired: 1 in, 2 out]
          n468 = TDMS Close(11:w572) -> ()  [unwired: 1 in, 2 out]
          n469 = TDMS Close(11:w570) -> ()  [unwired: 1 in, 2 out]
          n470 = TDMS Close(11:w569) -> ()  [unwired: 1 in, 2 out]
        }
      }
    }
    frame #2 {
      n471 = xnode "Read/Write Control"("FPGA VI Reference In"=w1174, "global stop"=TRUE) -> ("FPGA VI Reference Out"=w1173:refnum<k20>)  [unwired: 1 in, 1 out]
      n472 = xnode "Close FPGA VI Reference"("FPGA VI Reference In"=w1173) -> ()  [unwired: 1 in, 1 out]
    }
  }
  n473 = Open/Create/Replace File(file path (use dialog)=path "c:/methoden.per" ("Datei (Dialog verwenden)"), operation (0:open)=T3."open" ("Operation (0:Öffnen)")) -> (refnum out=w6:refnum<file>)  [unwired: 4 in, 2 out]
  n474 = Read from Binary File(5:T1 [] ("Methoden"), 11:w6) -> (2:w3:T1, 3:w5:refnum<file>)  [unwired: 4 in, 2 out]
  n475 = Close File(refnum=w5) -> ()  [unwired: 1 in, 2 out]
